vi "RT-Twosetup.vi"() -> ()   [LabVIEW 2015]
uses:
  <vilib>/Platform/TimedLoop/XDataNode/timing_clust.ctl
  <vilib>/Platform/TimedLoop/XDataNode/nitl_modes.ctl
  <vilib>/Platform/TimedLoop/XDataNode/wakeup.ctl
  <vilib>/Analysis/8numeric.llb/1D Numeric Integration.vi
  <vilib>/FPGAPlugInAG/myRIO-1900/niLvFpga_Open_myRIO-1900.vi
  <vilib>/rvi/interface/common/dynamic/niFpgaDynamicAddResources.vi
  <vilib>/Utility/error.llb/Error Cluster From Error Code.vi
  <vilib>/rvi/errors/niLvFpgaAdjustHostInterfaceError.vi
  <vilib>/RVI Host/nirviSupport.llb/nirviErrorClusterFromErrorCode.vi
  <vilib>/Analysis/3filter.llb/Butterworth Filter (DBL).vi
  <vilib>/FPGAPlugInAG/Dynamic/niLvFpga_Close_Dynamic.vi
  <vilib>/rvi/interface/nirviOpenFPGA/nirviOpenFPGA.xnode
  Ruichen Nov 5/FPGA Bitfiles/RuichenNov5_FPGATarget_FPGAWithLasertwo_aS1jXxUkL+g.lvbitx
  Ruichen Nov 5/FPGA_With Laser_twosetup_Jun15.vi
  <vilib>/rvi/interface/nirviReadWriteControl/nirviReadWriteControl.xnode
  <vilib>/Platform/TimedLoop/XDataNode/XDataNode.xnode
  <vilib>/rvi/interface/nirviMethod/nirviMethod.xnode
  <vilib>/rvi/interface/nirviCloseFPGA/nirviCloseFPGA.xnode
  NiFpgaLv.dll
  <vilib>/rvi/interface/Simulation/niFpgaSimulationCallBeginRW.vi
  <vilib>/rvi/interface/nirviMethod/StockFPGA_InlinedMethodWaitForSingleIRQ.vi
  <vilib>/FPGAPlugInAG/Dynamic/niLvFpga_WaitOnIrq_Dynamic.vi
  <vilib>/FPGAPlugInAG/Dynamic/niLvFpga_ReadFifo_Dynamic.vi
  <vilib>/rvi/errors/niLvFpgaMergeErrorWithErrorCode.vi
  <vilib>/FPGAPlugInAG/Dynamic/niLvFpga_AcknowledgeIrq_Dynamic.vi
  <vilib>/Analysis/NI_AALBase.lvlib
  <vilib>/Platform/TimedLoop/XDataNode/XDNodeRunTimeDep.lvlib
  <vilib>/Analysis/NI_AALPro.lvlib
  <vilib>/Analysis/NI_AAL_SigProc.lvlib
panel:
  in  "Gender 2":string="F"
  in  "Date 2":string="2015Aug1"
  in  "Fly # 2":i32=332
  in  "Filename Code 2":string="E1"
  in  "IRQ Bit (0-31) 2":u8
  in  "IRQ Bit (0-31)":u8
  in  "Double number of pixels to take per frame 2":u16=1536
  in  "Half-clocks between frames/Trigger frequency (us) 2":u16=1600
  in  "Half-clock time/FPGA loop timer(us) 2":u32=16
  in  "Gender":string="F"
  out "Raw Data":u16[](graph)=[289, 309, 323, 336, 353, 368, 382, 397, 412, 422, 437, 450, 463, 474, 485, 495, 506, 514, 526, 531, 540, 545, 552, 557, 563, 564, 568, 572, 575, 577, 580, 586, 587, 587, 592, 593, 596, 599, 601, 605, 607, 610, 611, 613, 618, 621, 625, 628, 629, 635, 636, 640, 643, 646, 649, 654, 656, 658, 660, 661, 664, 665, 669, 669, 673, 672, 674, 675, 677, 678, 681, 683, 684, 684, 686, 688, 688, 691, 691, 693, 694, 695, 697, 697, 699, 701, 702, 704, 709, 709, 711, 711, 713, 717, 721, 723, 726, 724, 728, 732, 734, 735, 738, 740, 743, 746, 750, 753, 754, 760, 763, 765, 769, 773, 774, 774, 774, 775, 774, 775, 775, 774, 776, 779, 780, 783, 781, 767, 792, 814, 820, 815, 817, 814, 815, 814, 814, 811, 810, 809, 807, 804, 802, 805, 803, 801, 801, 798, 799, 797, 797, 797, 797, 794, 795, 792, 791, 794, 791, 791, 792, 790, 790, 790, 789, 790, 790, 791, 792, 790, 792, 794, 793, 793, 795, 798, 796, 798, 797, 798, 799, 799, 801, 805, 803, 804, 804, 807, 808, 808, 811, 812, 815, 814, 816, 820, 819, 820, 822, 821, 823, 824, 823, 822, 822, 824, 825, 826, 826, 824, 827, 827, 828, 830, 830, 831, 830, 830, 828, 824, 820, 821, 817, 813, 813, 809, 807, 808, 805, 804, 802, 798, 798, 796, 795, 794, 793, 793, 791, 790, 791, 792, 788, 790, 789, 785, 787, 788, 788, 787, 788, 789, 789, 791, 793, 798, 722, 728, 740, 741, 746, 747, 750, 748, 753, 752, 757, 758, 761, 762, 767, 768, 768, 770, 775, 775, 776, 776, 781, 781, 785, 784, 787, 788, 792, 792, 794, 793, 798, 796, 795, 799, 800, 798, 799, 796, 797, 798, 802, 800, 805, 803, 806, 804, 808, 805, 810, 809, 812, 807, 808, 808, 812, 805, 806, 800, 803, 796, 798, 796, 800, 796, 798, 798, 800, 798, 800, 797, 799, 795, 794, 792, 793, 788, 789, 785, 788, 781, 785, 782, 785, 781, 782, 776, 778, 774, 772, 769, 770, 767, 769, 767, 764, 755, 755, 747, 747, 744, 743, 737, 737, 732, 732, 729, 728, 724, 723, 721, 720, 716, 718, 716, 717, 715, 721, 722, 724, 719, 718, 714, 715, 709, 710, 697, 718, 722, 731, 731, 727, 725, 722, 720, 718, 719, 718, 716, 714, 710, 705, 705, 703, 706, 704, 707, 708, 710, 712, 718, 720, 725, 726, 725, 728, 728, 724, 728, 726, 728, 725, 730, 732, 736, 735, 737, 734, 738, 737, 741, 742, 746, 743, 749, 747, 746, 745, 744, 743, 744, 746, 745, 747, 749, 748, 752, 754, 751, 752, 752, 749, 748, 748, 751, 752, 757, 758, 757, 757, 755, 756, 755, 753, 752, 749, 748, 746, 746, 744, 746, 744, 743, 739, 739, 740, 736, 735, 736, 733, 736, 737, 740, 736, 732, 729, 729, 726, 721, 716, 719, 717, 716, 713, 711, 706, 704, 699, 701, 698, 697, 697, 695, 692, 691, 687, 690, 684, 681, 679, 680, 674, 674, 668, 661, 690, 692, 694, 694, 692, 691, 692, 696, 694, 692, 694, 689, 691, 688, 690, 688, 689, 688, 690, 689, 688, 689, 689, 687, 689, 689, 690, 688, 689, 686, 687, 686, 685, 684, 683, 682, 683, 682, 682, 681, 681, 677, 677, 676, 677, 675, 674, 675, 674, 673, 670, 669, 670, 667, 667, 665, 664, 661, 659, 655, 656, 654, 655, 653, 651, 645, 643, 641, 642, 639, 638, 636, 637, 630, 630, 628, 627, 624, 623, 621, 620, 617, 616, 615, 614, 610, 610, 609, 606, 604, 606, 605, 604, 600, 600, 599, 598, 599, 600, 595, 597, 596, 597, 595, 595, 598, 598, 598, 599, 596, 593, 595, 597, 595, 597, 596, 596, 595, 599, 597, 596, 594, 594, 593, 592, 590, 593, 595, 638, 613, 615, 619, 622, 620, 622, 619, 622, 618, 619, 618, 621, 619, 621, 618, 622, 618, 618, 616, 615, 616, 617, 616, 621, 616, 618, 613, 615, 614, 612, 612, 615, 607, 610, 610, 610, 609, 610, 606, 607, 603, 604, 601, 601, 600, 604, 598, 600, 596, 599, 598, 600, 597, 598, 596, 597, 593, 595, 593, 597, 593, 595, 592, 593, 589, 591, 587, 589, 582, 585, 581, 582, 578, 581, 576, 573, 573, 570, 568, 570, 566, 565, 563, 563, 561, 558, 556, 557, 553, 550, 547, 545, 544, 540, 537, 537, 531, 529, 522, 523, 515, 514, 509, 506, 498, 493, 488, 482, 475, 468, 458, 454, 442, 436, 424, 419, 406, 397, 386, 378, 364, 353, 340, 330, 317, 308, 293]
  in  "FIFO Timeout setting (ms)":i32=5000
  out "Elements going into FIFO":u32=768
  in  "Wait on IRQ Timeout (ms)":i32=100
  in  "Stop LED illumination switch (permanant)":bool
  in  "sampling freq: fs":dbl=1000.0 format="%0.2f"
  in  "high cutoff freq: fh":dbl=400.0 format="%0.2f"
  in  "low cutoff freq: fl":dbl=40.0 format="%0.4f"
  in  "order":i32=3
  out "max index(es) of difference":i32=576
  in  "Threshhold position filter":i32=25
  out "Fly real-time location":dbl(graph)=575.5038458695241
  in  "Fly presence?":bool=TRUE
  in  "threshold 3":dbl=5.0
  out "slope/fly moving speed":dbl(graph)=2.647982912649468
  out "Fly real-time location/center mass":dbl(graph)=575.5038458695241
  in  "peaks/valleys":enum32{"Peaks", "Valleys"}(ring)
  in  "threshold":dbl format="%0.2f"
  out "Laser ON/OFF?":i16(graph)=1
  in  "Laser current control":u16=583
  in  "Laser current control 2":u16=629
  out "peak":i32(graph)=579
  in  "sampling freq: fs 1(2)":dbl=1000.0 format="%0.2f"
  in  "low cutoff freq: fl 1(2)":dbl=40.0 format="%0.4f"
  in  "order 1(2)":i32=3
  in  "Wait on IRQ Timeout (ms) 2":i32=100
  out "Raw Data 2":u16[](graph)=[263, 286, 311, 317, 343, 351, 376, 380, 406, 412, 436, 442, 466, 470, 490, 491, 513, 517, 533, 535, 551, 550, 570, 565, 584, 584, 596, 593, 610, 602, 616, 613, 625, 618, 629, 622, 634, 629, 640, 632, 641, 635, 645, 638, 651, 643, 653, 646, 656, 647, 658, 648, 659, 650, 660, 653, 665, 655, 667, 660, 673, 664, 674, 665, 678, 669, 683, 672, 681, 672, 684, 674, 684, 679, 687, 680, 692, 684, 697, 686, 699, 689, 703, 693, 706, 698, 711, 701, 710, 703, 717, 709, 718, 708, 719, 711, 725, 713, 723, 717, 731, 720, 730, 724, 737, 725, 737, 726, 738, 728, 737, 728, 741, 731, 741, 731, 736, 729, 737, 727, 737, 724, 734, 724, 730, 717, 721, 709, 709, 713, 719, 715, 721, 720, 724, 720, 727, 723, 726, 722, 730, 725, 727, 723, 725, 715, 721, 714, 719, 710, 715, 708, 715, 708, 711, 705, 712, 704, 707, 701, 704, 698, 705, 693, 698, 691, 696, 692, 693, 687, 691, 686, 694, 685, 693, 687, 692, 687, 692, 687, 690, 686, 692, 689, 694, 687, 692, 686, 694, 688, 692, 690, 697, 689, 699, 693, 699, 697, 704, 702, 709, 700, 709, 703, 708, 708, 713, 711, 720, 714, 720, 717, 722, 716, 722, 722, 729, 721, 728, 722, 729, 721, 727, 727, 730, 724, 730, 723, 728, 724, 730, 727, 730, 728, 734, 729, 736, 732, 741, 734, 745, 738, 748, 744, 750, 750, 757, 752, 760, 748, 757, 756, 761, 756, 753, 739, 782, 791, 792, 790, 786, 786, 786, 788, 786, 784, 785, 785, 786, 785, 786, 786, 786, 786, 789, 790, 793, 792, 796, 796, 799, 801, 801, 802, 806, 806, 806, 805, 806, 809, 811, 814, 818, 818, 823, 826, 827, 829, 831, 832, 835, 835, 837, 839, 839, 840, 843, 842, 843, 840, 840, 841, 841, 836, 836, 833, 832, 829, 826, 827, 826, 822, 824, 820, 817, 817, 817, 814, 816, 813, 813, 809, 807, 802, 802, 800, 797, 796, 799, 797, 798, 796, 797, 796, 801, 801, 803, 805, 809, 809, 809, 815, 812, 817, 816, 818, 822, 823, 824, 827, 826, 827, 832, 831, 832, 833, 834, 832, 830, 828, 831, 829, 827, 828, 827, 826, 827, 826, 826, 825, 823, 826, 827, 819, 808, 818, 814, 812, 802, 801, 796, 796, 790, 790, 786, 789, 784, 785, 781, 786, 782, 780, 777, 780, 777, 779, 776, 780, 775, 777, 775, 777, 769, 770, 767, 765, 760, 761, 756, 759, 753, 753, 748, 748, 743, 744, 739, 741, 737, 740, 737, 739, 731, 728, 726, 726, 720, 722, 716, 718, 713, 714, 708, 707, 703, 701, 698, 698, 695, 695, 692, 693, 687, 688, 685, 689, 685, 686, 682, 685, 684, 686, 684, 685, 682, 682, 680, 681, 679, 680, 677, 680, 677, 678, 678, 680, 677, 681, 679, 682, 679, 682, 682, 682, 681, 686, 684, 689, 690, 691, 690, 694, 692, 693, 694, 699, 696, 700, 698, 703, 702, 705, 704, 707, 706, 708, 706, 711, 708, 713, 713, 720, 663, 668, 673, 668, 674, 671, 673, 671, 675, 672, 674, 671, 674, 666, 671, 666, 669, 663, 667, 661, 666, 660, 662, 657, 658, 656, 655, 651, 655, 650, 653, 648, 649, 646, 648, 643, 646, 639, 646, 643, 644, 641, 643, 638, 643, 640, 642, 640, 646, 642, 645, 642, 647, 644, 645, 645, 648, 643, 649, 645, 646, 647, 650, 647, 647, 648, 650, 647, 650, 650, 653, 648, 653, 650, 654, 653, 657, 651, 656, 654, 657, 655, 659, 655, 659, 657, 659, 657, 660, 656, 660, 658, 663, 661, 664, 659, 665, 658, 665, 664, 668, 663, 668, 666, 671, 668, 673, 669, 671, 669, 675, 673, 675, 671, 677, 675, 676, 675, 677, 675, 678, 677, 677, 674, 679, 673, 671, 666, 670, 685, 676, 687, 678, 689, 680, 693, 681, 689, 679, 688, 678, 689, 677, 689, 677, 688, 674, 687, 674, 681, 674, 683, 671, 682, 672, 680, 668, 679, 666, 679, 667, 675, 663, 674, 663, 671, 661, 670, 662, 671, 660, 671, 659, 666, 654, 664, 651, 660, 649, 662, 651, 661, 650, 661, 651, 662, 650, 660, 654, 660, 654, 664, 653, 662, 657, 662, 653, 666, 652, 660, 656, 665, 653, 667, 657, 661, 652, 661, 646, 658, 646, 655, 642, 640, 614, 624, 630, 637, 629, 636, 625, 635, 624, 627, 617, 621, 611, 616, 604, 610, 596, 601, 587, 593, 579, 581, 566, 570, 554, 555, 537, 535, 515, 514, 494, 487, 467, 457, 437, 429, 406, 395, 375, 362, 339, 330]
  in  "FIFO Timeout setting (ms) 2":i32=5000
  in  "IRQ Number(s)":i32
  in  "high cutoff freq: fh 2(2)":dbl=400.0 format="%0.2f"
  in  "high cutoff freq: fh 2":dbl=400.0 format="%0.2f"
  in  "threshold 2":dbl=5.0
  out "Subtraction-10 frames average 2":dbl[](graph)=[-0.00376082484141181, -0.022873117346732395, -0.07050720237291398, -0.1540346374735344, -0.2738381122413475, -0.4232374215403344, -0.5915356082774301, -0.7649563748596452, -0.9279827571524178, -1.0689098028697672, -1.1818944407352858, -1.266468515907346, -1.3239301795845555, -1.3537298053317928, -1.3535024688465405, -1.3236736048293158, -1.2699765892033446, -1.196103151819737, -1.103481168748181, -0.9966608194463829, -0.8808932741469696, -0.7588132471338049, -0.6319358272774014, -0.5061901508981533, -0.389606531794253, -0.28341498123065917, -0.18402265448368677, -0.0895595758834902, -0.0008756313510866129, 0.07639693426695328, 0.133619958700495, 0.16938552040951854, 0.1903441584835061, 0.1997469061336739, 0.19643994001825865, 0.1826729540490901, 0.1615768169464919, 0.13332481872660476, 0.10013796877874595, 0.06705342198095826, 0.03830291760632126, 0.01812410505187573, 0.011040299585847513, 0.015678182445511897, 0.02081490655012259, 0.014702139724543097, -0.007694751105500634, -0.0446452896519642, -0.08670643610239012, -0.1277979715847761, -0.17541766675378068, -0.23978598654637842, -0.32345963765313057, -0.4259229913641579, -0.5469672931754658, -0.6838484323216937, -0.8312503325824077, -0.9825087887632742, -1.12867925796915, -1.2633122581370897, -1.388947954682801, -1.5076359517362217, -1.6119373954936247, -1.6958213101732502, -1.7616620044088953, -1.812529334752833, -1.8486816415803766, -1.8719732738452068, -1.8847414740848745, -1.8859257219554215, -1.8743803959335448, -1.849487948127098, -1.808197256512122, -1.7466329724933511, -1.6611929495136815, -1.5482907626170368, -1.4067508767371109, -1.238889497628028, -1.0483066610520457, -0.8410518480858593, -0.6285318110483396, -0.42486535833667716, -0.24156551097017567, -0.08552176857086577, 0.03983825028626295, 0.13356818406741786, 0.19717522191258308, 0.23278936634599218, 0.24150276211340116, 0.22730699422553458, 0.19899536076779312, 0.16605439722890952, 0.13693874170986747, 0.11613849442096771, 0.10209305304397168, 0.0912139405376808, 0.07866812938458467, 0.057773934292369024, 0.024749420335167242, -0.017230893747750352, -0.061913083640327604, -0.10784179345245254, -0.15830391148879083, -0.2143877330715396, -0.276778621610512, -0.3528272911072182, -0.44913895643011553, -0.5595612194406266, -0.6704730509504452, -0.7745604578629908, -0.8731593145809257, -0.9701116617591585, -1.069496797609171, -1.1730905057698047, -1.2777684274273855, -1.379916659751327, -1.4814777777037755, -1.588047949586358, -1.6986990178288548, -1.802015100812946, -1.8826514219000368, -1.9293015986204978, -1.9402172728964677, -1.9208181943344855, -1.8769697908343117, -1.8134710392918705, -1.733963461335194, -1.638587583967085, -1.523674399142967, -1.386346749941397, -1.2291419386239086, -1.0583515986225247, -0.8836878074942338, -0.7187385558367253, -0.5738173894502159, -0.45542305080593687, -0.3701037445479088, -0.317616230630637, -0.28930799633113535, -0.27602190239510177, -0.27115275142298206, -0.2717125476718229, -0.2774216061797233, -0.2867771895763348, -0.2981017950239787, -0.31178072131091655, -0.32608937059191756, -0.3353603508176363, -0.3357385368030959, -0.32681389734130667, -0.31103915970614604, -0.2946481407676892, -0.2807293154814101, -0.26451167744311843, -0.2407094121827115, -0.211050327886528, -0.1837625411526074, -0.16707239135883667, -0.16611371302420752, -0.18394775224048487, -0.21857278595226554, -0.2612999759586515, -0.30543475903423317, -0.35471060592599035, -0.41718212157458284, -0.49648878909719873, -0.5921132750867147, -0.7022809147875497, -0.825066949533824, -0.9576931927650932, -1.0951203986321776, -1.2307248788941316, -1.3591314014615774, -1.47693568696294, -1.5800230024344128, -1.6623793299744725, -1.719229265770608, -1.748876372099362, -1.7497891567424408, -1.7174342402814031, -1.6478702779804903, -1.5444577832306738, -1.4177442273018168, -1.280676739644643, -1.1434442501256068, -1.0128407801542985, -0.8932081460963361, -0.7801274495106644, -0.6621789141760148, -0.5372155137010306, -0.416657868348343, -0.31038743641522437, -0.21810966155455125, -0.13683865247976046, -0.06492287746215691, 0.0011107561638208675, 0.061355697754530085, 0.11016677649880281, 0.14364453618861886, 0.15949885750470377, 0.15778587381061385, 0.14364154198124413, 0.1227551498373353, 0.10305638615350414, 0.09370311790900986, 0.09640586325429953, 0.1068123624264574, 0.12066322960728416, 0.13426468214309775, 0.1405369170182361, 0.13235826724673255, 0.11110335132503889, 0.08002488785588409, 0.03737629353642087, -0.018637808401881423, -0.08700059597261785, -0.16054846664987324, -0.23088586621000848, -0.3000360164872003, -0.3758296150061959, -0.46236970350596185, -0.5587974369384311, -0.660898934677404, -0.7660448460774516, -0.8729260247349662, -0.9767431951499936, -1.0748340624377097, -1.1705342177905071, -1.2675451899107062, -1.3683321205241692, -1.4704192038160353, -1.5635451916548424, -1.6386695835358795, -1.693256497574253, -1.7277824542414204, -1.7420870638626291, -1.7322894565104652, -1.6933942206714316, -1.624322634361078, -1.528407672990961, -1.4124576261429136, -1.2832747700098635, -1.1468778581044203, -1.01116382986234, -0.8850483573844115, -0.7788370742693432, -0.7004306032861471, -0.6487688874247476, -0.6180821163401873, -0.6030060400253653, -0.5959037847747308, -0.5875920612480976, -0.5741500995988539, -0.5582423972416175, -0.5439443648942461, -0.5328073893976564, -0.5232639086012941, -0.5146518432728002, -0.5090998137587567, -0.5065819566515576, -0.5038548193517427, -0.5005796544437178, -0.5002479504085452, -0.5014087461956691, -0.495040446888778, -0.4727119725533419, -0.43125038067469823, -0.3715074504347726, -0.3008338507948245, -0.23340738667639166, -0.17755289527540508, -0.13118575191904772, -0.09305928514965348, -0.06698996053837801, -0.058563480577701686, -0.07181350001125919, -0.10793573000127399, -0.1689908845929966, -0.25596119116887905, -0.3615529177179252, -0.4739173690044841, -0.5852687043626082, -0.6925790166307004, -0.7935196446787861, -0.8831899624548932, -0.9549489633523359, -1.0053936034989386, -1.034287291347867, -1.0417180668143775, -1.0307381755818692, -1.0022200877051664, -0.9517839735970008, -0.8847816574868836, -0.8203025453751498, -0.7740566015333439, -0.7450169971868286, -0.7211422986874927, -0.695447400598044, -0.6662409751476156, -0.6267691166515336, -0.5709534536668012, -0.5062730580488137, -0.4485965248982422, -0.4042914265127707, -0.36774155042836065, -0.3351346131083027, -0.31079122745476945, -0.29983578466573796, -0.29704845614316383, -0.28648550431823483, -0.2560797219170984, -0.207191797964983, -0.15002634485714278, -0.0941146339452417, -0.04141132907327572, 0.00732382089288372, 0.04527845665160592, 0.06729656650068232, 0.07648330949975393, 0.08064998018063296, 0.08649692634618564, 0.09611867663977593, 0.10592138239814952, 0.11046023397899403, 0.10860213666725135, 0.10263107983657813, 0.0951675648597761, 0.08755686894783427, 0.07727335537096702, 0.06050473908625864, 0.03858170245257776, 0.019016774014489195, 0.006217689491663469, -0.004829580964054308, -0.02187946084338151, -0.05041171001791412, -0.09262496242405108, -0.14569587160812036, -0.20561733612433442, -0.27547542848413525, -0.364110224847606, -0.4722816750400199, -0.5869343272139628, -0.6915599909578858, -0.7801941030271669, -0.856503792838089, -0.9183491975010316, -0.9560750231796934, -0.9649909582222269, -0.9473373048466116, -0.9066887049224265, -0.846911733740316, -0.7719296640245625, -0.6853692031922703, -0.5898590863699504, -0.4838455537247155, -0.3599201532402052, -0.20883433515499233, -0.028636455612853818, 0.16983555954076301, 0.36973615220851197, 0.5591901850809423, 0.733067351126909, 0.8883202563929481, 1.0221095816515888, 1.1375825701281228, 1.2453575621607862, 1.3512137702495255, 1.452792799750593, 1.5477941475302321, 1.6378527323460585, 1.729241387236583, 1.824010182307176, 1.9170375875927546, 2.0097098629114285, 2.108943976314938, 2.215027391713627, 2.3230331304401033, 2.429548985942421, 2.5355477549070238, 2.6464477153608295, 2.7702576533997356, 2.9131377100839217, 3.073678261038705, 3.244552757581614, 3.4204261801800553, 3.602300947020557, 3.794056055282762, 3.996592870664724, 4.2075413784439135, 4.424550583066579, 4.648714283923216, 4.880038620061748, 5.110417378684536, 5.330743067375148, 5.538073955911634, 5.732219184144099, 5.918123480846642, 6.110372500362169, 6.327000370177558, 6.583321692370052, 6.8906167476800295, 7.255257453715437, 7.68027948763792, 8.166604119726658, 8.712237640790278, 9.313494022979661, 9.964056663838145, 10.654892015352061, 11.378324058152502, 12.127175033359443, 12.895230216622453, 13.678603979404247, 14.474046709861591, 15.279470627616204, 16.090738173396232, 16.902158085596497, 17.714679222144923, 18.53315978571027, 19.358338660702593, 20.187216642994212, 21.01194814379528, 21.82222777219512, 22.61602191722952, 23.400763975924672, 24.184327855534672, 24.971785834110076, 25.768504552430322, 26.57753306161372, 27.396165036084163, 28.221325795503553, 29.049922125954453, 29.873139470742423, 30.679593833577684, 31.4609081749663, 32.212712825571906, 32.933051665490176, 33.619965819210464, 34.271625765457, 34.8890859732, 35.478764581385875, 36.04756436585725, 36.596346257203344, 37.12343236422261, 37.626822539780484, 38.105588462364175, 38.56611234545378, 39.01491060125615, 39.44715283367774, 39.853534247824754, 40.2310712889892, 40.57888757186952, 40.892349191698884, 41.16933128074967, 41.414110482177485, 41.63342646341003, 41.83363247239842, 42.018303435619615, 42.18872817010225, 42.34408970348531, 42.47754928608451, 42.58236130365064, 42.65971748760769, 42.713644181365986, 42.74525521883325, 42.748753326527726, 42.713333823695294, 42.63449439250565, 42.51642043459606, 42.364574210563276, 42.17993378111193, 41.9556039072654, 41.68122828230601, 41.35096432259596, 40.962156501385, 40.512861591872834, 40.00642312420001, 39.451821047297614, 38.85541134665982, 38.2173537339134, 37.53692246110689, 36.813455534636056, 36.044893402993836, 35.2315962369416, 34.377010210901396, 33.484762597643936, 32.557001280199344, 31.593345539691676, 30.589708555804926, 29.540802457970848, 28.44559042107734, 27.307847611971, 26.133341471138614, 24.926617171868227, 23.690992747103518, 22.429412137004675, 21.141197570572455, 19.823253456474465, 18.472937657505387, 17.085399392921254, 15.65521449602104, 14.180158509493307, 12.661336060618844, 11.104659392517387, 9.520123594285872, 7.917416475572328, 6.3027034652523515, 4.682263341486394, 3.0660056719976527, 1.4612989176075901, -0.13139771239858228, -1.7123880812285628, -3.2751905848703613, -4.808174608992262, -6.297740620268804, -7.7271473935905215, -9.081790002488592, -10.356133616169028, -11.554151135074896, -12.685676557678587, -13.758362721441806, -14.77575035037717, -15.74255078525408, -16.666415835412305, -17.556443863742437, -18.41732773000568, -19.24820734880522, -20.050495274673978, -20.828771105634228, -21.584545223346325, -22.314638216729037, -23.014595247144705, -23.680923116221063, -24.31176928795577, -24.907986296652496, -25.472415693796478, -26.006884426442767, -26.509208132203728, -26.97444501410167, -27.398008728417842, -27.77647645316585, -28.110048905215564, -28.40385378205497, -28.668367565302646, -28.917474740737617, -29.15755911012913, -29.384038238726703, -29.589748868420692, -29.76924544606401, -29.918328165454806, -30.036045206361063, -30.12937311357554, -30.208794995708473, -30.277806917764497, -30.332825573826625, -30.37151391821005, -30.39725409536827, -30.412656938396555, -30.413956258287868, -30.39735109458483, -30.36367151738291, -30.31652542478745, -30.261502338976612, -30.204184510465918, -30.14871940232551, -30.097352108584346, -30.047784376662662, -29.993910764165935, -29.92747733828788, -29.837193104698244, -29.711437717836816, -29.54242404233223, -29.327043752160268, -29.067452267851255, -28.771375859675317, -28.448234996158785, -28.103706205315063, -27.739064252815734, -27.354938800750066, -26.95410602345842, -26.539649974551562, -26.111747453405904, -25.670224697083718, -25.216450073218372, -24.750712831780145, -24.272616690419394, -23.78091619861165, -23.2753928522925, -22.761343164505224, -22.244816004276867, -21.72786594335049, -21.21417978538097, -20.71071063748661, -20.222789714979534, -19.753607797772467, -19.301867144951565, -18.86158004391697, -18.43123343688248, -18.0143840109354, -17.61041314054533, -17.212941896681723, -16.81748076620043, -16.426715057545632, -16.04531884239273, -15.675168217712752, -15.31754391861577, -14.974344529674788, -14.649051560367349, -14.343674232203869, -14.054821664391083, -13.777985913802734, -13.508879451605642, -13.242082589313352, -12.97275008446546, -12.696082444150797, -12.409256262549752, -12.112442043542092, -11.807571599785787, -11.503046705893926, -11.21227271056884, -10.942267303072779, -10.691045639568582, -10.457244745998056, -10.244016574854548, -10.051518531924048, -9.87061623279275, -9.685855538473072, -9.483993882353875, -9.258017630799372, -9.007354147311343, -8.735371178658298, -8.443853548820478, -8.134648990461866, -7.813610715699731, -7.487832383457061, -7.162206460899759, -6.839682212706416, -6.5231322433607275, -6.217234714158364, -5.9289138057546955, -5.6619823667673765, -5.412579923126114, -5.173133122357569, -4.938792509122974, -4.710971908054537, -4.495125783066928, -4.29488827490601, -4.109283009973048, -3.9339855929532987, -3.764175462971437, -3.5958951815680615, -3.4233935393454833, -3.2394830683479725, -3.044598200547575, -2.8492028556439815, -2.6649359565198165, -2.498850507216461, -2.351994989596593, -2.2200416457008263, -2.097354106644154, -1.9816741134997693, -1.8733763519173783, -1.7695976868323733, -1.6661986077487314, -1.5661702552726366, -1.4769612407021504, -1.4022436450621427, -1.3413180588193816, -1.2916765418291913, -1.2507505025842343, -1.217944653778875, -1.1955330573680045, -1.1903154857303306, -1.2136419659976456, -1.2738107603937543, -1.3724390980490855, -1.507885962350215, -1.6763896973186003, -1.8711191364837378, -2.080717766297735, -2.2916512250453622, -2.4928182004627035, -2.6755849779817424, -2.831334628203854, -2.949936208348438, -3.018931043968457, -3.0298384774615834, -2.986716161838226, -2.9013396647233263, -2.783940766628996, -2.6407616499493893, -2.4767875282446816, -2.3001157310922586, -2.119033148960194, -1.9363683567416965, -1.753289795851237, -1.5770678151434212, -1.4153899237661798, -1.26683678826652, -1.1294693920602856, -1.0081263553709296, -0.9063889971623248, -0.8232096500754797, -0.7569594986576507, -0.7051277446235275, -0.6609626172844825, -0.616778811364658, -0.5706830022030382, -0.5238540351402355, -0.47530875658731897, -0.42318424546559685, -0.3665577694236487, -0.30756730783451597, -0.252067836451747, -0.20443771113836468, -0.16562044808556212, -0.13522655672247405, -0.11042486682504797, -0.08882597340265397, -0.07538417283274809, -0.07845722411255573, -0.09901308223776047, -0.13026897814939803, -0.167681023057152, -0.216864963214016, -0.2876508278340629, -0.3808876121771616, -0.48834768637964654, -0.6016077538625505, -0.7144036890985765, -0.8233041134798268, -0.9286804831666096, -1.0311741155510397, -1.1278050469591983, -1.21391289217402, -1.2898718155112867, -1.3623238656310392, -1.4395570531631365, -1.525478966414576, -1.6149241061519883, -1.6997189909924915, -1.778996289119347, -1.856765587267083, -1.9288164466428759, -1.9803244023449569, -1.9995236930547802, -1.9845766247298668, -1.9402420483774412, -1.8734661368225516, -1.7868241836145662, -1.678066806724053, -1.5470606760189267, -1.3999431271868326, -1.2465844830197161, -1.0965471302864371, -0.9576500186057677, -0.8342253141905895, -0.7249247595230404, -0.6233497672777235, -0.5244663209042256, -0.43092374400637523, -0.34844608354784923, -0.27579555458255645, -0.205640126840743, -0.13310105896139204, -0.05745891472761272, 0.020014086631217332, 0.09599766173239417]
  out "Integral of fly movement 2":dbl(graph)=79328.12499999988
  out "Fly real-time location/center mass 2":dbl(graph)=449.3915049700411
  in  "Fly presence? 2":bool=TRUE
  in  "Threshhold position filter 2":i32=25
  out "Subtraction-10 frames average":dbl[](graph)=[-0.00017411226117643476, -0.0013055996545707524, -0.0035903395574269233, -0.006140247965520452, -0.00923276869863789, -0.014513306411590609, -0.024099157253657542, -0.039967772567530944, -0.06357541427301813, -0.09583108984311303, -0.13590150060754386, -0.18222853004778936, -0.23497195652311498, -0.29627873859507925, -0.36762235578800867, -0.4458020453794083, -0.5236122536857144, -0.5933213778936878, -0.6504861464069396, -0.6979211584984373, -0.7411188663256683, -0.7815085830005122, -0.8183155891766691, -0.8521623071897098, -0.8841462084502619, -0.9134837246856654, -0.9369680551554314, -0.9497776612221199, -0.9486128151755009, -0.9320974118038038, -0.8980743313625289, -0.8467722222222394, -0.7831903740903514, -0.7091535422572258, -0.6191326605534678, -0.5096162410693632, -0.38445407095366013, -0.25038829684524394, -0.11278151470849465, 0.027599357220651342, 0.17105909212912457, 0.31047378816969246, 0.43477068100652727, 0.5404159738124296, 0.6300372451091932, 0.7028022222295014, 0.755728962675972, 0.7909826153091774, 0.8173402496662823, 0.8426901249940745, 0.8646090232247912, 0.8743645244461501, 0.8649039706505928, 0.8319565719228973, 0.7750164581136465, 0.6955035375961216, 0.595281511328262, 0.47813554162155286, 0.34852361101846857, 0.21192255735328513, 0.07591841420380419, -0.05221188114593133, -0.1699837988889325, -0.28130279822899423, -0.39034428199093896, -0.4976048670003517, -0.600986712631866, -0.6958495060431942, -0.776729298015907, -0.8400889448088852, -0.886367229474972, -0.9177076114860692, -0.9344855611862907, -0.9368525887383509, -0.9256879281616348, -0.9041394572607666, -0.8777818783736817, -0.8490193014663585, -0.8164059788053225, -0.7777460019674792, -0.7306702277622628, -0.6758164055484195, -0.6196815773574544, -0.5696251531398948, -0.5294590057849148, -0.5036816824661907, -0.4967820810630079, -0.5075400503507222, -0.5296116117376369, -0.5541794866502316, -0.572591220019981, -0.5770013677344076, -0.5579969792703307, -0.5077796604374197, -0.42865181791737544, -0.33090735363867285, -0.22215393525511828, -0.10432496528395577, 0.023095326221807485, 0.15705894844325297, 0.2880394188853618, 0.40439012577347405, 0.4963650319027993, 0.5611047944479498, 0.6048704375837946, 0.6333678585164843, 0.6444899475696537, 0.6328680620173739, 0.5949073615035211, 0.5317088662054599, 0.4484691112083726, 0.35262691347111735, 0.25592435302870753, 0.1677918630477906, 0.08552896387664585, 0.001721814571532223, -0.08465072369990116, -0.16887968342886978, -0.2446520248995666, -0.3085125998395212, -0.36285963309259667, -0.412304954070232, -0.45947045202927694, -0.5043419236517144, -0.5430792956503917, -0.5701392528804239, -0.5823970562876603, -0.5798838911637391, -0.5657644118110517, -0.5445993018003239, -0.5216310512058843, -0.5004822604773764, -0.48152211922137, -0.46657488631796473, -0.45829805549562763, -0.45812891230711617, -0.46688057094727364, -0.4832346439961762, -0.5040900061989401, -0.5246298701963221, -0.5396268618306358, -0.5486879364347477, -0.5553220286350682, -0.5602243690739389, -0.5619992550807327, -0.5616390340191147, -0.5618614340001415, -0.5619878499927449, -0.556044076174116, -0.5375776201240388, -0.5018226807722814, -0.4441251771537087, -0.3609544857301398, -0.2542849281294559, -0.1337061514028871, -0.01077592265797097, 0.10802739138302234, 0.2204702742907546, 0.32334046947867695, 0.41151196363946524, 0.4802339911288074, 0.5261902901839506, 0.5468284379398634, 0.5388710085338079, 0.5013551052040558, 0.4402253796787686, 0.3649945548717722, 0.28453393264954674, 0.20500115403415162, 0.12737052447350872, 0.0491965117891805, -0.033624099556903625, -0.12401511839311359, -0.21772721743544826, -0.30600877804536525, -0.3845380193961243, -0.45271563684577065, -0.5083720110481487, -0.5483993223855057, -0.5692595973559456, -0.5689429763761056, -0.5496008669456361, -0.515240588241775, -0.47411449414621015, -0.43757582550721474, -0.4100771941058324, -0.3912010975889608, -0.3827420386611698, -0.3870110616763467, -0.4048639535633476, -0.43620163141685364, -0.4793177697728358, -0.5289343816851729, -0.5783732084027549, -0.6226483831393546, -0.659195235246784, -0.6900328665239266, -0.717743997948285, -0.7393052243940111, -0.7488387052387162, -0.7410064339076299, -0.7151668280354428, -0.6795465516096135, -0.6411676626175322, -0.5963042174390132, -0.5382989954290448, -0.4642086308424046, -0.3750273950060304, -0.27666264335898244, -0.1726805762033885, -0.061141495920442324, 0.055284462096357824, 0.16923993804278972, 0.2757778422982206, 0.3702189250517674, 0.44567248716703034, 0.4961833944600499, 0.519491459859946, 0.5161197856703529, 0.48925516442404415, 0.4457811453867938, 0.3931640243514122, 0.335508631703314, 0.27666000462165524, 0.22536122034470552, 0.18892461638725597, 0.16561938458101683, 0.14877029060355898, 0.1316923262868149, 0.10936359529509165, 0.07708080345845039, 0.03176571652430371, -0.02126415203944002, -0.07462865099459134, -0.12787029966300012, -0.18232016801891016, -0.23903213138123067, -0.3005074000846957, -0.36721761077858145, -0.4351648227660777, -0.49748480603309386, -0.5504691500712211, -0.5969563855516151, -0.6388566462772594, -0.6732204448166237, -0.6957500128580998, -0.704492654543993, -0.7053606511252234, -0.7068255505670542, -0.7111454456488149, -0.7171014427168811, -0.7204222977914532, -0.7121147912086817, -0.682707841299486, -0.6275912533817392, -0.5508914834780626, -0.4629445080600611, -0.374231847988499, -0.29348756884376326, -0.22608532636693335, -0.1717419914367267, -0.12418215830144208, -0.0759240199102344, -0.023465854733136317, 0.03495613368073635, 0.10364757933210111, 0.186875978170696, 0.28047176945614266, 0.37246623408448487, 0.4537540089905635, 0.5221189090366725, 0.5772629148585383, 0.6195437842721869, 0.6505398797841452, 0.6673383091587535, 0.6621500666273517, 0.6294188669879256, 0.5678884026793507, 0.4776367246700199, 0.3619901254764424, 0.22990267247159088, 0.09066434134522192, -0.04648363107378383, -0.16799140274521498, -0.2619477892108051, -0.3288086467882362, -0.3780169598975864, -0.4147345107790823, -0.4399946988218713, -0.45778196758191586, -0.4728903322312472, -0.48932022274099063, -0.5119453113587404, -0.5438949360668957, -0.5850957300740083, -0.6332562764482668, -0.6817369661192783, -0.7196211852955186, -0.7411725102754282, -0.7520087863705485, -0.7603886734107392, -0.7693352686888594, -0.7780724435008916, -0.7860412698523446, -0.7953131974335302, -0.8093398039386801, -0.8283695763831367, -0.8473220299068974, -0.8630717050367799, -0.8783577081132093, -0.892945116030908, -0.8982166970622634, -0.8843691812454313, -0.8489983341041851, -0.7981453240654648, -0.7378847051244974, -0.6655070232853431, -0.5735742180168014, -0.45708106421106715, -0.31639925961468957, -0.1590737866558735, 0.0033355840614780405, 0.16185921651742433, 0.31258646062391215, 0.452338343404292, 0.5749805575018252, 0.6712888680367465, 0.7315341547033588, 0.7517398814338361, 0.7348880070093617, 0.6857398390731334, 0.6111385134913258, 0.5228723096640573, 0.4318324111699806, 0.34025172401448045, 0.24736937305364776, 0.15784156635128652, 0.07651042206858172, 0.003772883581942832, -0.0629782232996971, -0.1286940081175351, -0.19772726178007713, -0.2713596192561732, -0.34779592456603625, -0.42333992685501454, -0.49628751054437203, -0.5666772253075136, -0.6286643732283865, -0.6728023696181352, -0.6962315973004579, -0.703034713648139, -0.7020136014256354, -0.703404439937798, -0.710015320364523, -0.7156617656943353, -0.7127960782972558, -0.6987305516219793, -0.6767153962682136, -0.6525149153664662, -0.6316849293158644, -0.6187483363957781, -0.6144729279978336, -0.6180486050640402, -0.6330864189293007, -0.6627772041805703, -0.7019166712317585, -0.7393755374665935, -0.765505461453525, -0.7764222036847284, -0.7696638037044172, -0.74111805905735, -0.6910322911182983, -0.623579160676762, -0.5383420920997759, -0.43065265289455934, -0.3002573308746692, -0.15092259425682136, 0.015622110790919387, 0.1946442614540931, 0.3730903109812267, 0.5367123338443216, 0.6790157566567216, 0.7995832395645845, 0.8951896619070442, 0.9608299845005637, 0.9968364468122866, 1.0067579713827326, 0.9912086432745015, 0.9482471263296486, 0.8811804893600276, 0.7989187264121542, 0.7078954125144599, 0.6120374936386584, 0.5141496232828386, 0.4142079445676434, 0.31468652890071547, 0.22211899540161129, 0.1399216579039876, 0.07005059700724892, 0.017247963468361452, -0.015501622682586178, -0.03254984006910774, -0.04612893264658296, -0.06952650175657003, -0.11252353348731638, -0.18040885529329365, -0.2721680628995837, -0.3822515911818568, -0.5017857806819399, -0.6198988731614818, -0.7262369995249518, -0.8111728656936505, -0.8684225357345006, -0.8990058995890593, -0.9075499623628133, -0.8977470496940952, -0.8745268143081815, -0.8441468656929902, -0.8112598244140514, -0.778277057340187, -0.7477741175043585, -0.7252892407870994, -0.7168386207607349, -0.7232909271474866, -0.7365659877890743, -0.7414056214816782, -0.7280969588471254, -0.7004614128383602, -0.6670127989797451, -0.6331576747915737, -0.5977492527834072, -0.5524997568983321, -0.4900541210242786, -0.40608708648086494, -0.29564160282918805, -0.15660928933041263, 0.007186595218111103, 0.18629507602397022, 0.36646272580965705, 0.5332396031733194, 0.6768763941517248, 0.7907893517687489, 0.8712917590344003, 0.922780189304281, 0.9537929539711842, 0.9687394176061441, 0.9693260986597775, 0.9552998439742726, 0.9240374691005266, 0.8771673370192855, 0.8211939500761857, 0.7591571431502234, 0.6926676856627026, 0.6284730370506213, 0.5707184781226731, 0.5152431462804957, 0.45636062097298347, 0.3918646995312176, 0.32210119515646674, 0.24777271899974834, 0.16944111121942207, 0.08427298985578352, -0.013485790267639703, -0.12456713336305435, -0.24399633307965893, -0.3642314265649915, -0.4747812371557585, -0.5646437823813745, -0.6265764327719912, -0.6573275140072035, -0.6558789526974032, -0.6221897569890409, -0.5600029777218457, -0.4804061725317835, -0.3934102515117905, -0.30283676942819754, -0.21228827793009214, -0.12333279093058303, -0.035098823919149306, 0.04911526715647138, 0.12628668299424806, 0.20141522088447067, 0.280948100266101, 0.3626726363188982, 0.4384522788136301, 0.5061083683109453, 0.575375006200826, 0.6582532028795898, 0.7558580451840798, 0.8603507020065457, 0.9653936278157114, 1.0692725123865725, 1.1718470525300688, 1.272738426840291, 1.3709577035007996, 1.4661433723369786, 1.559081041169027, 1.6489409903984935, 1.731769923726097, 1.801486773489075, 1.8537182263756429, 1.8902753234771437, 1.9186485003323326, 1.9460313929763289, 1.97442918741, 2.0056475617894116, 2.0446506904852857, 2.092528372086769, 2.1483396284249947, 2.215650396354458, 2.294876136594476, 2.381207065473582, 2.4748699018686904, 2.579717423360695, 2.698160537409042, 2.8323892111726123, 2.9816208879989032, 3.1442066260393498, 3.324402132118785, 3.5261056451825965, 3.746273498221313, 3.9836396532216556, 4.242440972110447, 4.5259197205480985, 4.834539532183516, 5.168294180188352, 5.52727552599602, 5.907827657991055, 6.304448282685934, 6.717446041575664, 7.150231908029313, 7.603695367024238, 8.077557189762695, 8.569383573295394, 9.073002597804843, 9.586155756115309, 10.116177716337475, 10.674086352879788, 11.269313159769121, 11.907593760086048, 12.58596064564858, 13.293872665342972, 14.021698080945395, 14.760652096041209, 15.498437700869376, 16.22492798636594, 16.939702787230615, 17.653266946601153, 18.381937914543425, 19.134436194857358, 19.902814424794155, 20.67064045169619, 21.424507186952862, 22.15791275844625, 22.872347661912087, 23.573707576768765, 24.264767732228037, 24.940021340560794, 25.588797898169314, 26.202635937391022, 26.776155442184255, 27.306843522461016, 27.79660513139952, 28.250350047289217, 28.672709014652686, 29.064973148731724, 29.42510629441868, 29.751221359110012, 30.04682421891593, 30.319605834762413, 30.57308847323303, 30.80819053733222, 31.03032226851724, 31.244481307843223, 31.44860922606201, 31.633219821591105, 31.785118037096588, 31.894683720978225, 31.95779661586935, 31.971838584533376, 31.93230113062428, 31.83445047092844, 31.679985300967314, 31.47904662556253, 31.240073211247434, 30.9618103917683, 30.641239024952768, 30.281875468623436, 29.889428407606488, 29.465243368494367, 29.010043956957578, 28.52972296658352, 28.029754915590125, 27.509353290472298, 26.96514906445715, 26.39317290784618, 25.788417105068145, 25.149083022013173, 24.476259573025132, 23.768571743932227, 23.025287939120506, 22.251106424242593, 21.450648124554377, 20.622293136463593, 19.761151721111734, 18.865577196239634, 17.940123139596853, 16.990428329916373, 16.018388105591544, 15.026700188156017, 14.01436384300455, 12.97083500677785, 11.889881275078858, 10.77466922188803, 9.628258702052682, 8.454448195724423, 7.265133695016243, 6.076365535034785, 4.893365123282578, 3.7095532614713296, 2.517763517138069, 1.3140267408770159, 0.10309209642734382, -1.097192432889481, -2.267385411930342, -3.3944907621586125, -4.469239206666381, -5.489787294397093, -6.459802537068538, -7.38100261281204, -8.257687685899288, -9.100751446659293, -9.922390196002823, -10.73071732580621, -11.5262653960874, -12.302138094129747, -13.051669492570305, -13.771894442454053, -14.458721932895862, -15.108005691893894, -15.72129731761331, -16.307379747694846, -16.877187908027814, -17.43744317765741, -17.991119943063904, -18.54065018507351, -19.08674531756916, -19.62278622788451, -20.13463627958771, -20.60680191243237, -21.02438534875431, -21.376310849903668, -21.658624268879443, -21.86977992174831, -22.011941620880712, -22.09505301916887, -22.129394797421718, -22.123365749377168, -22.08586833329003, -22.020104554291713, -21.9238000455441, -21.79858267495767, -21.653175725941942, -21.498289904431616, -21.343914968258687, -21.197799477152486, -21.062728377100974, -20.938961251530145, -20.824718023521243, -20.717206642785232, -20.615462348219484, -20.515811184705363, -20.412387296008212, -20.30451311016455, -20.194590015757164, -20.082154952053266, -19.965437180049225, -19.84418363236728, -19.71966080590015, -19.59101651633682, -19.451896747520415, -19.29630570606669, -19.124625370339928, -18.940908553959353, -18.74841398094579, -18.548334850520973, -18.34390884585281, -18.142670376332994, -17.946870545009805, -17.74763036520624, -17.535438988826193, -17.309111329506337, -17.073475808836182, -16.838228485832403, -16.616666753603663, -16.416761917507017, -16.237902387884915, -16.077044504285908, -15.927991530686892, -15.778194878136429, -15.618016239883016, -15.44547675943471, -15.259036731177005, -15.057565030108478, -14.841515625944622, -14.608958358145568, -14.358650294416119, -14.09462865748661, -13.822698270104837, -13.54650548098001, -13.265495449822433, -12.973379194579834, -12.6637392519324, -12.336642526018718, -11.99750459600148, -11.654793828507898, -11.314946313361293, -10.97644226630489, -10.635343587106952, -10.290828574749673, -9.944251504563086, -9.601837487332826, -9.273690255644487, -8.967830376318314, -8.689646700736837, -8.443309094072085, -8.230419468928783, -8.049589622644953, -7.899441492653072, -7.778172513279259, -7.678654073677392, -7.588666634736229, -7.496717485742737, -7.397547046258119, -7.289718378538725, -7.168077924542731, -7.028490811396077, -6.877623118566651, -6.7283616982472125, -6.588994662979143, -6.45961051981716, -6.335907389209561, -6.213871508147667, -6.092452979069016, -5.972482269112145, -5.853392865729774, -5.732945383951386, -5.606896264537465, -5.469907708842971, -5.322011725262907, -5.170622617466721, -5.019133870887847, -4.861231237999979, -4.6918455000478305, -4.51214993000221, -4.324497437985056, -4.131660461805229, -3.9392579288830207, -3.754622884073377, -3.5851706825546588, -3.4381831491227537, -3.3172911818944666, -3.219947302195386, -3.138072117665304, -3.059582753466284, -2.9724515330751533, -2.869044637751715, -2.7454704463662214]
  out "Elements going into FIFO 2":u32=768
  out "peak 2":i32(graph)=455
  out "Locations":dbl[](array[numeric])=[578.761004094259, 639.2528301043833, 668.0679203678199, 696.7815537364846, 725.476037300267, 754.2154459301402]
  out "size(s) 2":i32=7
  out "Peak":dbl=579.0
  out "Locations 2":dbl[](array[numeric])=[464.590182599329, 527.8415122083895, 556.6315016603198, 585.3519264680052, 614.0835380602954, 642.7960329445821, 671.488231054549]
  out "y":dbl
  out "size(s)":i32=6
  out "Peak 2":dbl=455.0
  out "Wait on IRQ Timed Out?":bool
  out "Frame Count":i16=10040
  out "Wait on IRQ Timed Out? 2":bool
  in  "Stop FPGA data acquisition":bool
  in  "high cutoff freq: fh 1(2)":dbl=400.0 format="%0.2f"
  in  "Manual control for laser":bool
  in  "sampling freq: fs 2(2)":dbl=1000.0 format="%0.2f"
  in  "low cutoff freq: fl 2(2)":dbl=40.0 format="%0.4f"
  in  "order 2(2)":i32=3
  in  "sampling freq: fs 2":dbl=1000.0 format="%0.2f"
  in  "low cutoff freq: fl 2":dbl=40.0 format="%0.4f"
  in  "order 2":i32=3
  in  "threshold 4":dbl format="%0.2f"
  in  "peaks/valleys 2":enum32{"Peaks", "Valleys"}(ring)
  out "x/y 2":dbl=449.3915049700411
  out "x/y":dbl=575.5038458695241
  out "Subtraction-10 frames average (threshold and flipped)":dbl[](graph)=[0.0, 0.0, 0.0, 0.0, 0.0, 0.0, 0.0, 0.0, 0.0, 0.0, 0.0, 0.0, 0.0, 0.0, 0.0, 0.0, 0.0, 0.0, 0.0, 0.0, 0.0, 0.0, 0.0, 0.0, 0.0, 0.0, 0.0, 0.0, 0.0, 0.0, 0.0, 0.0, 0.0, 0.0, 0.0, 0.0, 0.0, 0.0, 0.0, 0.0, 0.0, 0.0, 0.0, 0.0, 0.0, 0.0, 0.0, 0.0, 0.0, 0.0, 0.0, 0.0, 0.0, 0.0, 0.0, 0.0, 0.0, 0.0, 0.0, 0.0, 0.0, 0.0, 0.0, 0.0, 0.0, 0.0, 0.0, 0.0, 0.0, 0.0, 0.0, 0.0, 0.0, 0.0, 0.0, 0.0, 0.0, 0.0, 0.0, 0.0, 0.0, 0.0, 0.0, 0.0, 0.0, 0.0, 0.0, 0.0, 0.0, 0.0, 0.0, 0.0, 0.0, 0.0, 0.0, 0.0, 0.0, 0.0, 0.0, 0.0, 0.0, 0.0, 0.0, 0.0, 0.0, 0.0, 0.0, 0.0, 0.0, 0.0, 0.0, 0.0, 0.0, 0.0, 0.0, 0.0, 0.0, 0.0, 0.0, 0.0, 0.0, 0.0, 0.0, 0.0, 0.0, 0.0, 0.0, 0.0, 0.0, 0.0, 0.0, 0.0, 0.0, 0.0, 0.0, 0.0, 0.0, 0.0, 0.0, 0.0, 0.0, 0.0, 0.0, 0.0, 0.0, 0.0, 0.0, 0.0, 0.0, 0.0, 0.0, 0.0, 0.0, 0.0, 0.0, 0.0, 0.0, 0.0, 0.0, 0.0, 0.0, 0.0, 0.0, 0.0, 0.0, 0.0, 0.0, 0.0, 0.0, 0.0, 0.0, 0.0, 0.0, 0.0, 0.0, 0.0, 0.0, 0.0, 0.0, 0.0, 0.0, 0.0, 0.0, 0.0, 0.0, 0.0, 0.0, 0.0, 0.0, 0.0, 0.0, 0.0, 0.0, 0.0, 0.0, 0.0, 0.0, 0.0, 0.0, 0.0, 0.0, 0.0, 0.0, 0.0, 0.0, 0.0, 0.0, 0.0, 0.0, 0.0, 0.0, 0.0, 0.0, 0.0, 0.0, 0.0, 0.0, 0.0, 0.0, 0.0, 0.0, 0.0, 0.0, 0.0, 0.0, 0.0, 0.0, 0.0, 0.0, 0.0, 0.0, 0.0, 0.0, 0.0, 0.0, 0.0, 0.0, 0.0, 0.0, 0.0, 0.0, 0.0, 0.0, 0.0, 0.0, 0.0, 0.0, 0.0, 0.0, 0.0, 0.0, 0.0, 0.0, 0.0, 0.0, 0.0, 0.0, 0.0, 0.0, 0.0, 0.0, 0.0, 0.0, 0.0, 0.0, 0.0, 0.0, 0.0, 0.0, 0.0, 0.0, 0.0, 0.0, 0.0, 0.0, 0.0, 0.0, 0.0, 0.0, 0.0, 0.0, 0.0, 0.0, 0.0, 0.0, 0.0, 0.0, 0.0, 0.0, 0.0, 0.0, 0.0, 0.0, 0.0, 0.0, 0.0, 0.0, 0.0, 0.0, 0.0, 0.0, 0.0, 0.0, 0.0, 0.0, 0.0, 0.0, 0.0, 0.0, 0.0, 0.0, 0.0, 0.0, 0.0, 0.0, 0.0, 0.0, 0.0, 0.0, 0.0, 0.0, 0.0, 0.0, 0.0, 0.0, 0.0, 0.0, 0.0, 0.0, 0.0, 0.0, 0.0, 0.0, 0.0, 0.0, 0.0, 0.0, 0.0, 0.0, 0.0, 0.0, 0.0, 0.0, 0.0, 0.0, 0.0, 0.0, 0.0, 0.0, 0.0, 0.0, 0.0, 0.0, 0.0, 0.0, 0.0, 0.0, 0.0, 0.0, 0.0, 0.0, 0.0, 0.0, 0.0, 0.0, 0.0, 0.0, 0.0, 0.0, 0.0, 0.0, 0.0, 0.0, 0.0, 0.0, 0.0, 0.0, 0.0, 0.0, 0.0, 0.0, 0.0, 0.0, 0.0, 0.0, 0.0, 0.0, 0.0, 0.0, 0.0, 0.0, 0.0, 0.0, 0.0, 0.0, 0.0, 0.0, 0.0, 0.0, 0.0, 0.0, 0.0, 0.0, 0.0, 0.0, 0.0, 0.0, 0.0, 0.0, 0.0, 0.0, 0.0, 0.0, 0.0, 0.0, 0.0, 0.0, 0.0, 0.0, 0.0, 0.0, 0.0, 0.0, 0.0, 0.0, 0.0, 0.0, 0.0, 0.0, 0.0, 0.0, 0.0, 0.0, 0.0, 0.0, 0.0, 0.0, 0.0, 0.0, 0.0, 0.0, 0.0, 0.0, 0.0, 0.0, 0.0, 0.0, 0.0, 0.0, 0.0, 0.0, 0.0, 0.0, 0.0, 0.0, 0.0, 0.0, 0.0, 0.0, 0.0, 0.0, 0.0, 0.0, 0.0, 0.0, 0.0, 0.0, 0.0, 0.0, 0.0, 0.0, 0.0, 0.0, 0.0, 0.0, 0.0, 0.0, 0.0, 0.0, 0.0, 0.0, 0.0, 0.0, 0.0, 0.0, 0.0, 0.0, 0.0, 0.0, 0.0, 0.0, 0.0, 0.0, 0.0, 0.0, 0.0, 0.0, 0.0, 0.0, 0.0, 0.0, 0.0, 0.0, 0.0, 0.0, 0.0, 0.0, 0.0, 0.0, 0.0, 0.0, 0.0, 0.0, 0.0, 0.0, 0.0, 0.0, 0.0015670103505882691, 0.009835162018197504, 0.029616981315390506, 0.0625014042989501, 0.1128672492615259, 0.18893829900662376, 0.29738855173323925, 0.44223295825623055, 0.6266176323046234, 0.8530721043548897, 1.1195086267764147, 1.4210912037033385, 1.7579488476005198, 2.132581663522992, 2.5443857111810946, 2.9911684792637425, 3.468324330744002, 3.967399669097878, 4.483873119162557, 5.022939628251187, 5.593678904351159, 6.203838755444227, 6.857755021041721, 7.551353240776067, 8.273270190466423, 9.013315955611118, 9.762381248785578, 10.508042346645308, 11.240204913753823, 11.958602176812073, 12.673976795087388, 13.402935642992084, 14.154512006459548, 14.921071503776977, 15.68647722967134, 16.437586723403527, 17.168123865894394, 17.879761827917736, 18.578535061483343, 19.267315509630166, 19.94065485107036, 20.587907926490743, 21.20061134804935, 21.773362012470162, 22.303608716104222, 22.793208356915386, 23.247017737729212, 23.669613741528863, 24.062235930611784, 24.42280126710537, 24.749382026038226, 25.045450584475503, 25.318671827800443, 25.57254918261367, 25.80798889748239, 26.030394943548952, 26.24476362311442, 26.449039082604603, 26.633740599884508, 26.785680551654124, 26.895247326618097, 26.958329591603263, 26.97231793349423, 26.932711936450882, 26.83478494473758, 26.680241640654486, 26.47922779272328, 26.240185712318198, 25.96186313058943, 25.641242275096147, 25.281839996437817, 24.88936476166169, 24.465161338335747, 24.009952193974744, 23.52962875232784, 23.02966405787837, 22.50927012482069, 21.965076537470125, 21.393112719774017, 20.78836989048062, 20.14904855006249, 19.476236951774425, 18.768559616432118, 18.025284662101672, 17.251110223283675, 16.4506572222573, 15.622305852443837, 14.761166544450004, 13.865592832437217, 12.940138535050163, 11.990442677515443, 11.018400835304778, 10.026710946448254, 9.018377046715681, 7.993209335224144, 6.955237075219014, 5.918833408849362, 4.905527908146546, 3.938882350810046, 3.040910829708238, 2.2297850167548834, 1.5185773006845253, 0.9148116840918452, 0.42061396168423154, 0.033277641146948075, -0.25391101488384754, -0.45071787436917377, -0.5689777740820747, -0.6216598772948659, -0.6220350118161854, -0.5829782423007939, -0.5164229367698447, -0.4329689102945371, -0.34163679474788267, -0.24975337699672212, -0.1629479501462467, -0.08523734797621368, -0.0191768624275769, 0.033944746396776505, 0.07388585532560793, 0.10122512116673613, 0.11714092258053928, 0.12320759321881623, 0.1212157781470316, 0.1130213522923148, 0.10042482109888484, 0.08508104144793928, 0.06843747802508315, 0.05169803812773066, 0.03580877401874596, 0.021461357353519072, 0.009110155824285256, -0.0010010856369361914, -0.008806601489307852, -0.01438316394706807, -0.017914458859385547, -0.019657322877674833, -0.019911326791130717, -0.018992672289735762, -0.017212912718820476, -0.014862624556584781, -0.012199850624656991, -0.009442908173550974, -0.006767000432727104, -0.004303981359620368, -0.0021445905669832356, -0.0003424881511090148, 0.0010805334093793217, 0.0021287113054894273, 0.0028263126637286615, 0.0032118437454117035, 0.003332745205073464, 0.0032407621363534055, 0.0029880982276751784, 0.002624395387240247, 0.0021945249467137805, 0.0017371342931631014, 0.001283862999172809, 0.0008591241265219373, 0.00048033787999283864, 0.00015850447162665864, -0.00010099086962094713, -0.00029743709498482676, -0.000433803365069504, -0.0005157592291269795, -0.0005507605895506344, -0.0005472379875448193, -0.0005139099450998233, -0.0004592320798930045, -0.00039098275090484536, -0.00031597819430329114, -0.00023990442937639526, -0.00016724950178684773, -0.00010131765849671445, -4.430654083164826e-05, 2.5708563599211424e-06, 3.8936176272048425e-05, 6.508222935043747e-05, 8.180817306000358e-05, 9.026285139125543e-05, 9.18032440302056e-05, 8.787259352768435e-05, 7.990066868139865e-05, 6.922684156872292e-05, 5.7045230912518924e-05, 4.4370096602770004e-05, 3.2018939970799924e-05, 2.0610337949553413e-05, 1.0573373197966623e-05, 2.16556830155219e-06, -4.503559198638388e-06, -9.445880576292187e-06, -1.2767143033843909e-05, -1.4640296044249864e-05, -1.5280961949059467e-05, -1.4925947354422648e-05, -1.3815323628844693e-05, -1.2178288493994586e-05, -1.0222762504495106e-05, -8.128475708787543e-06, -6.0431588612096455e-06, -4.0813653543798535e-06, -2.325407828765382e-06, -8.278893798237667e-07, 3.846647960387457e-07, 1.3075216719983282e-06, 1.9531847587151984e-06, 2.346882858354879e-06, 2.5223454965963513e-06, 2.5180377119313567e-06, 2.373963016215043e-06, 2.1290875201931016e-06, 1.819391782633431e-06, 1.4765204108781223e-06, 1.1269726649244673e-06, 7.917596351974685e-07, 4.864439527247501e-07, 2.214752015170936e-07, 2.7368833971454915e-09, -1.6777242423565418e-07, -2.911914656684078e-07, -3.7103873545350995e-07, -4.1248947989521215e-07, -4.217200289414555e-07, -4.0534120772317083e-07, -3.699327881554181e-07, -3.2168264893914156e-07, -2.6612764931772895e-07, -2.0798820007495557e-07, -1.510850521629356e-07, -9.832476777581503e-08, -5.173949418667696e-08, -1.256680656270379e-08, 1.8643704948562634e-08, 4.1908975919676554e-08, 5.768621337892809e-08, 6.674996284383223e-08, 7.007863209795617e-08, 6.87547215918295e-08, 6.388130534203529e-08, 5.6515835377881136e-08, 4.762113731982407e-08, 3.80325332412121e-08, 2.8439362005429538e-08, 1.937874528207435e-08, 1.1239239047963183e-08, 4.271979974447629e-09, -1.392953978888771e-09, -5.7270363828919865e-09, -8.782424705409298e-09, -1.0671199320762074e-08]
  out "Integral of fly movement":dbl(graph)=46937.50000197561
  out "Subtraction-10 frames average (threshold and flipped) 2":dbl[](graph)=[0.0, 0.0, 0.0, 0.0, 0.0, 0.0, 0.0, 0.0, 0.0, 0.0, 0.0, 0.0, 0.0, 0.0, 0.0, 0.0, 0.0, 0.0, 0.0, 0.0, 0.0, 0.0, 0.0, 0.0, 0.0, 0.0, 0.0, 0.0, 0.0, 0.0, 0.0, 0.0, 0.0, 0.0, 0.0, 0.0, 0.0, 0.0, 0.0, 0.0, 0.0, 0.0, 0.0, 0.0, 0.0, 0.0, 0.0, 0.0, 0.0, 0.0, 0.0, 0.0, 0.0, 0.0, 0.0, 0.0, 0.0, 0.0, 0.0, 0.0, 0.0, 0.0, 0.0, 0.0, 0.0, 0.0, 0.0, 0.0, 0.0, 0.0, 0.0, 0.0, 0.0, 0.0, 0.0, 0.0, 0.0, 0.0, 0.0, 0.0, 0.0, 0.0, 0.0, 0.0, 0.0, 0.0, 0.0, 0.0, 0.0, 0.0, 0.0, 0.0, 0.0, 0.0, 0.0, 0.0, 0.0, 0.0, 0.0, 0.0, 0.0, 0.0, 0.0, 0.0, 0.0, 0.0, 0.0, 0.0, 0.0, 0.0, 0.0, 0.0, 0.0, 0.0, 0.0, 0.0, 0.0, 0.0, 0.0, 0.0, 0.0, 0.0, 0.0, 0.0, 0.0, 0.0, 0.0, 0.0, 0.0, 0.0, 0.0, 0.0, 0.0, 0.0, 0.0, 0.0, 0.0, 0.0, 0.0, 0.0, 0.0, 0.0, 0.0, 0.0, 0.0, 0.0, 0.0, 0.0, 0.0, 0.0, 0.0, 0.0, 0.0, 0.0, 0.0, 0.0, 0.0, 0.0, 0.0, 0.0, 0.0, 0.0, 0.0, 0.0, 0.0, 0.0, 0.0, 0.0, 0.0, 0.0, 0.0, 0.0, 0.0, 0.0, 0.0, 0.0, 0.0, 0.0, 0.0, 0.0, 0.0, 0.0, 0.0, 0.0, 0.0, 0.0, 0.0, 0.0, 0.0, 0.0, 0.0, 0.0, 0.0, 0.0, 0.0, 0.0, 0.0, 0.0, 0.0, 0.0, 0.0, 0.0, 0.0, 0.0, 0.0, 0.0, 0.0, 0.0, 0.0, 0.0, 0.0, 0.0, 0.0, 0.0, 0.0, 0.0, 0.0, 0.0, 0.0, 0.0, 0.0, 0.0, 0.0, 0.0, 0.0, 0.0, 0.0, 0.0, 0.0, 0.0, 0.0, 0.0, 0.0, 0.0, 0.0, 0.0, 0.0, 0.0, 0.0, 0.0, 0.0, 0.0, 0.0, 0.0, 0.0, 0.0, 0.0, 0.0, 0.0, 0.0, 0.0, 0.0, 0.0, 0.0, 0.0, 0.0, 0.0, 0.0, 0.0, 0.0, 0.0, 0.0, 0.0, 0.0, 0.0, 0.0, 0.0, 0.0, 0.0, 0.0, 0.0, 0.0, 0.0, 0.0, 0.0, 0.0, 0.0, 0.0, 0.0, 0.0, 0.0, 0.0, 0.0, 0.0, 0.0, 0.0, 0.0, 0.0, 0.0, 0.0, 0.0, 0.0, 0.0, 0.0, 0.0, 0.0, 0.0, 0.0, 0.0, 0.0, 0.0, 0.0, 0.0, 0.0, 0.0, 0.0, 0.0, 0.0, 0.0, 0.0, 0.0, 0.0, 0.0, 0.0, 0.0, 0.0, 0.0, 0.0, 0.0, 0.0, 0.0, 0.0, 0.0, 0.0, 0.0, 0.0, 0.0, 0.0, 0.0, 0.0, 0.0, 0.0, 0.0, 0.0, 0.0, 0.0, 0.0, 0.0, 0.0, 0.0, 0.0, 0.0, 0.0, 0.0, 0.0, 0.0, 0.0, 0.0, 0.0, 0.0, 0.0, 0.0, 0.0, 0.0, 0.0, 0.0, 0.0, 0.0, 0.0, 0.0, 0.0, 0.0, 0.0, 0.0, 0.0, 0.0, 0.0, 0.0, 0.0, 0.0, 0.0, 0.0, 0.0, 0.0, 0.0, 0.002507216560941266, 0.015666614324645556, 0.048414529367267235, 0.10313440140338344, 0.17806738457215382, 0.27638400615030273, 0.40850251946819616, 0.5826561862390891, 0.8008618061615357, 1.0653420537211697, 1.374836621626359, 1.7162886000050817, 2.073775278150525, 2.442047707571892, 2.8262619457227838, 3.2332631070768025, 3.6638833247839324, 4.1136951734422835, 4.579809216262396, 5.064560309861075, 5.571264949596996, 6.095727468266008, 6.62812785721717, 7.1635834482372625, 7.702333598059364, 8.240753530099408, 8.771971617054342, 9.296659141199958, 9.824764622439657, 10.366485706278588, 10.92791780350326, 11.512804570909568, 12.12125987778636, 12.746511131548859, 13.378984827940439, 14.012759197101206, 14.644809431979695, 15.274947129931881, 15.908813105263839, 16.550924294039927, 17.197230457061497, 17.843374114517147, 18.48851003277664, 19.130558547899923, 19.771000532000166, 20.417111106324278, 21.075941039014047, 21.749986513010082, 22.437472533298543, 23.13639088145387, 23.844792525523793, 24.559886291371047, 25.280428260286897, 26.009447289427165, 26.755456335369214, 27.52723984130693, 28.326338457814444, 29.147237324104637, 29.984786306320444, 30.835579270324367, 31.690676129152138, 32.536063628333835, 33.359065546718305, 34.14927245379277, 34.897299434386625, 35.59546833315736, 36.23847089177154, 36.822675376943465, 37.34857469647627, 37.822502506534164, 38.249212490939925, 38.62591571145494, 38.948660038589445, 39.22057263619253, 39.45050075826299, 39.646533528351895, 39.81284096272003, 39.95183728361499, 40.06374034836224, 40.1427461259492, 40.18177498996225, 40.17789685256884, 40.130245076296205, 40.037948478777665, 39.901557298089, 39.72642950926712, 39.519874781389866, 39.28320140062926, 39.00776666080765, 38.67973564878157, 38.290036945837116, 37.83863753465352, 37.33001742712581, 36.765885899438324, 36.14446487636626, 35.46651384981923, 34.73684375147922, 33.95978011138459, 33.137666816599136, 32.27278097572319, 31.368467369173967, 30.430622800968795, 29.46546101901217, 28.471160275386435, 27.439228633408575, 26.366710984784408, 25.257914605641524, 24.1165739819294, 22.945198165127387, 21.751653818211928, 20.548157779647365, 19.342432544257157, 18.134251221825792, 16.917539596906334, 15.683205954797899, 14.423595619519771, 13.136084554575138, 11.819644378242469, 10.473415312568882, 9.105397955106326, 7.737250162256155, 6.399218995122498, 5.123550865904613, 3.9399204295022847, 2.872536212783016, 1.9385967771303432, 1.1477941520232, 0.5025902011410339, -0.0009751299881771841, -0.3721488848055948, -0.6241720459243078, -0.7729611035089212, -0.8358633182195697, -0.8305542848186875, -0.7741198332640722, -0.6823420345204461, -0.5691912287058133, -0.4465124490780447, -0.32388507713625614, -0.2086285979186188, -0.10592441105227426, -0.019023231227144097, 0.05049088374432922, 0.10240594768529054, 0.13757918671595867, 0.15764393311998295, 0.1647399305767762, 0.16127650625935747, 0.14973423537378766, 0.13250740449472775, 0.11178684900975283, 0.08948062348416182, 0.06716844712493636, 0.046084904138771955, 0.027125903624754137, 0.010872835891032592, -0.002370883512064254, -0.01253569883065571, -0.019738394948350526, -0.024234603368385534, -0.02637399808531339, -0.02656010274857497, -0.025215945026465333, -0.022756191767973246, -0.019565894551659038, -0.01598557581877214, -0.012302090107452415, -0.008744496454637495, -0.005484066345455407, -0.0026375136774829753, -0.0002725548393658878, 0.0015850262232665468, 0.002943534901660944, 0.0038373545858983865, 0.004319251556597223, 0.004453355842469689, 0.0043090605150068175, 0.003955976995729938, 0.0034599945548559625, 0.0028804198536812667, 0.002268117395202728, 0.0016645333382224623, 0.0011014617804312613, 0.000601402300797686, 0.00017835796526951238, -0.00016106825319188016, -0.0004164059403924115, -0.0005919872933464482, -0.0006956429012188081, -0.0007374904600494944, -0.0007288635657819155, -0.0006814094723785729, -0.0006063688685042619, -0.0005140376658841887, -0.00041340062147396427, -0.00031191926326144077, -0.00021545184324920505, -0.00012828058973076917, -5.3221003759286174e-05, 8.211054453049759e-06, 5.5596608505313514e-05, 8.939435854054577e-05, 0.00011072091226774912, 0.00012114285994809677, 0.00012248969322173299, 0.00011669341219954827, 0.00010565788111035373, 9.115865344046231e-05, 7.477212528641314e-05, 5.783148909708864e-05, 4.14060213844254e-05, 2.6299700706527097e-05, 1.3064957532522651e-05, 2.0274405917046533e-06, -6.682021068039328e-06, -1.3091638109814746e-05, -1.7351907059344366e-05, -1.970015197328063e-05, -2.042805665804812e-05, -1.985334042705061e-05, -1.829624379725893e-05, -1.6061074324428943e-05, -1.3422724650516662e-05, -1.0617816413894041e-05, -7.839941765416986e-06, -5.238362082905027e-06, -2.9194719213185884e-06, -9.503347541570801e-07, 6.363653394380072e-07, 1.8365459530496355e-06, 2.668628190405467e-06, 3.1675297327907646e-06, 3.3790646530444027e-06, 3.354972973859355e-06, 3.1487184509922794e-06, 2.812119499958635e-06, 2.3928172657262186e-06, 1.9325371668130534e-06, 1.4660655610317025e-06, 1.0208405463435474e-06, 6.170439263936521e-07, 2.680783503956665e-07, -1.8682232820305408e-08, -2.409711989004527e-07, -4.0062624662619165e-07, -5.025788780146264e-07, -5.538944954686978e-07, -5.629055640556186e-07, -5.384656971340867e-07, -4.893396039238219e-07, -4.237329407920402e-07, -3.4895739556821744e-07, -2.7121980983432905e-07, -1.9551968850687653e-07, -1.2563685055518215e-07, -6.418997299279064e-08, -1.274707579640505e-08, 2.8029715293981596e-08, 5.8220799922373366e-08, 7.84803734373567e-08, 8.987295153535555e-08, 9.372312281232547e-08, 9.14839999227371e-08, 8.462758503413809e-08, 7.455832932507073e-08, 6.254958701913161e-08, 4.970145124067221e-08, 3.691759865297685e-08, 2.4898232423841318e-08, 1.4145957166592797e-08, 4.981397159258544e-09, -2.434470058871928e-09, -8.073998170208512e-09, -1.2014926023003749e-08, -1.441272344669942e-08, -1.547470982627999e-08, -1.5436999700990535e-08, -1.4544938476142128e-08, -1.3037349626558023e-08, -1.1134630681566902e-08, -9.03051194543155e-09, -6.887128367119495e-09, -4.832947142684552e-09, -2.9630352161644768e-09, -1.3411341758993554e-09, -3.026819906756002e-12, 1.0392784488925986e-09, 1.792960134158715e-09, 2.2797385935177352e-09, 2.5314457416114777e-09, 2.5860095935717633e-09, 2.4839862944067344e-09, 2.265712344314631e-09, 1.969098988006786e-09, 1.6280499899374264e-09, 1.2714533330667787e-09, 9.226762456483308e-10, 5.994804469677418e-10, 3.142694017538793e-10, 7.45803296982467e-11, -1.1626066223867908e-10, -2.5839301715849153e-10, -3.5464740271049003e-10, -4.0979225763171095e-10, -4.2983870024450915e-10, -4.214297350151918e-10, -3.913292455903789e-10, -3.460172603624e-10, -2.9139060298004885e-10, -2.3256234713666333e-10, -1.7374942887500608e-10, -1.182351979115691e-10, -6.839242529119728e-11, -2.5752109474012255e-11, 8.89589434625133e-12, 3.538308419973726e-11, 5.40342930970579e-11, 6.554041681256562e-11, 7.083883525270828e-11, 7.100650830828549e-11, 6.716891707229812e-11, 6.042643443548774e-11, 5.179838467411166e-11, 4.218400567728285e-11, 3.233875679286564e-11, 2.28639020776352e-11, 1.4207014748837311e-11, 6.670959024058489e-12, 4.2897231841655177e-13, -4.456344381456035e-12, -8.0120536737751e-12, -1.0333536984810293e-11, -1.1564053006380647e-11, -1.1876141923834467e-11, -1.1455506389740646e-11, -1.0487722227573808e-11, -9.147895635722496e-12, -7.593193169851863e-12, -5.9580265436031064e-12, -4.351574133697137e-12, -2.857260851987012e-12, -1.5337922873835503e-12, -4.1734154148082527e-13, 4.754884130156259e-13, 1.144263936714131e-12, 1.601168519613736e-12, 1.8675311721543142e-12, 1.9706115945405574e-12, 1.940764988302127e-12, 1.8090609820145927e-12, 1.6053892928910144e-12, 1.357050329386041e-12, 1.087802236170644e-12, 8.173166782054621e-13, 5.60983369697872e-13, 3.2999713413385193e-13, 1.316601380104397e-13, -3.016518548300851e-14, -1.5451116491552708e-13, -2.4271868651056814e-13, -2.9785163740987455e-13, -3.241445767776164e-13, -3.2650715192975674e-13, -3.10100403811924e-13, -2.799927389151506e-13, -2.408971723970767e-13, -1.9698655040656087e-13, -1.5177982991170486e-13, -1.0809005429054997e-13, -6.802328578500155e-14, -3.301728350886168e-14, -3.908974322425524e-15, 1.8979422608282268e-14, 3.5744556555249506e-14, 4.6803895982623886e-14, 5.280143758356358e-14, 5.4521611740523173e-14, 5.281438283838379e-14, 4.8533254026853485e-14, 4.248678672771646e-14, 3.5403354925950423e-14, 2.790817658541066e-14, 2.0511190247658236e-14, 1.3604055518789669e-14, 7.464426990592305e-15, 2.265653963981411e-15, -1.9098362054412302e-15, -5.055033831300829e-15, -7.222057262756574e-15, -8.506161944938648e-15, -9.030875755245517e-15, -8.934842205765206e-15, -8.360729018605128e-15]
  out "Fly real-time location 2":dbl(graph)=449.3915049700411
  out "max index(es) of difference 2":i32=449
  out "slope/fly moving speed 2":dbl(graph)=6.524815642372175
  out "s? t:f":dbl=1.0
  out "Laser ON/OFF? 2":i16(graph)=1
  out "Iteration Duration":i64=50
  out "sum":dbl
  in  "Date":string="2015Aug1"
  in  "Fly #":i32=331
  in  "Filename Code":string="E1"
  in  "LED High Period (ticks)":u32=1520
  in  "Apply":bool=TRUE
  in  "Output Enable":bool=TRUE
  in  "LED High Period (ticks) 2":u32=615
  in  "Apply 2":bool=TRUE
  in  "Output Enable 2":bool=TRUE
  out "FIFO Timed Out?":bool
  out "FIFO Timed Out? 2":bool
  in  "Double number of pixels to take per frame":u16=1536
  in  "Half-clocks between frames/Trigger frequency (us)":u16=1600
  in  "Half-clock time/FPGA loop timer(us)":u32=16
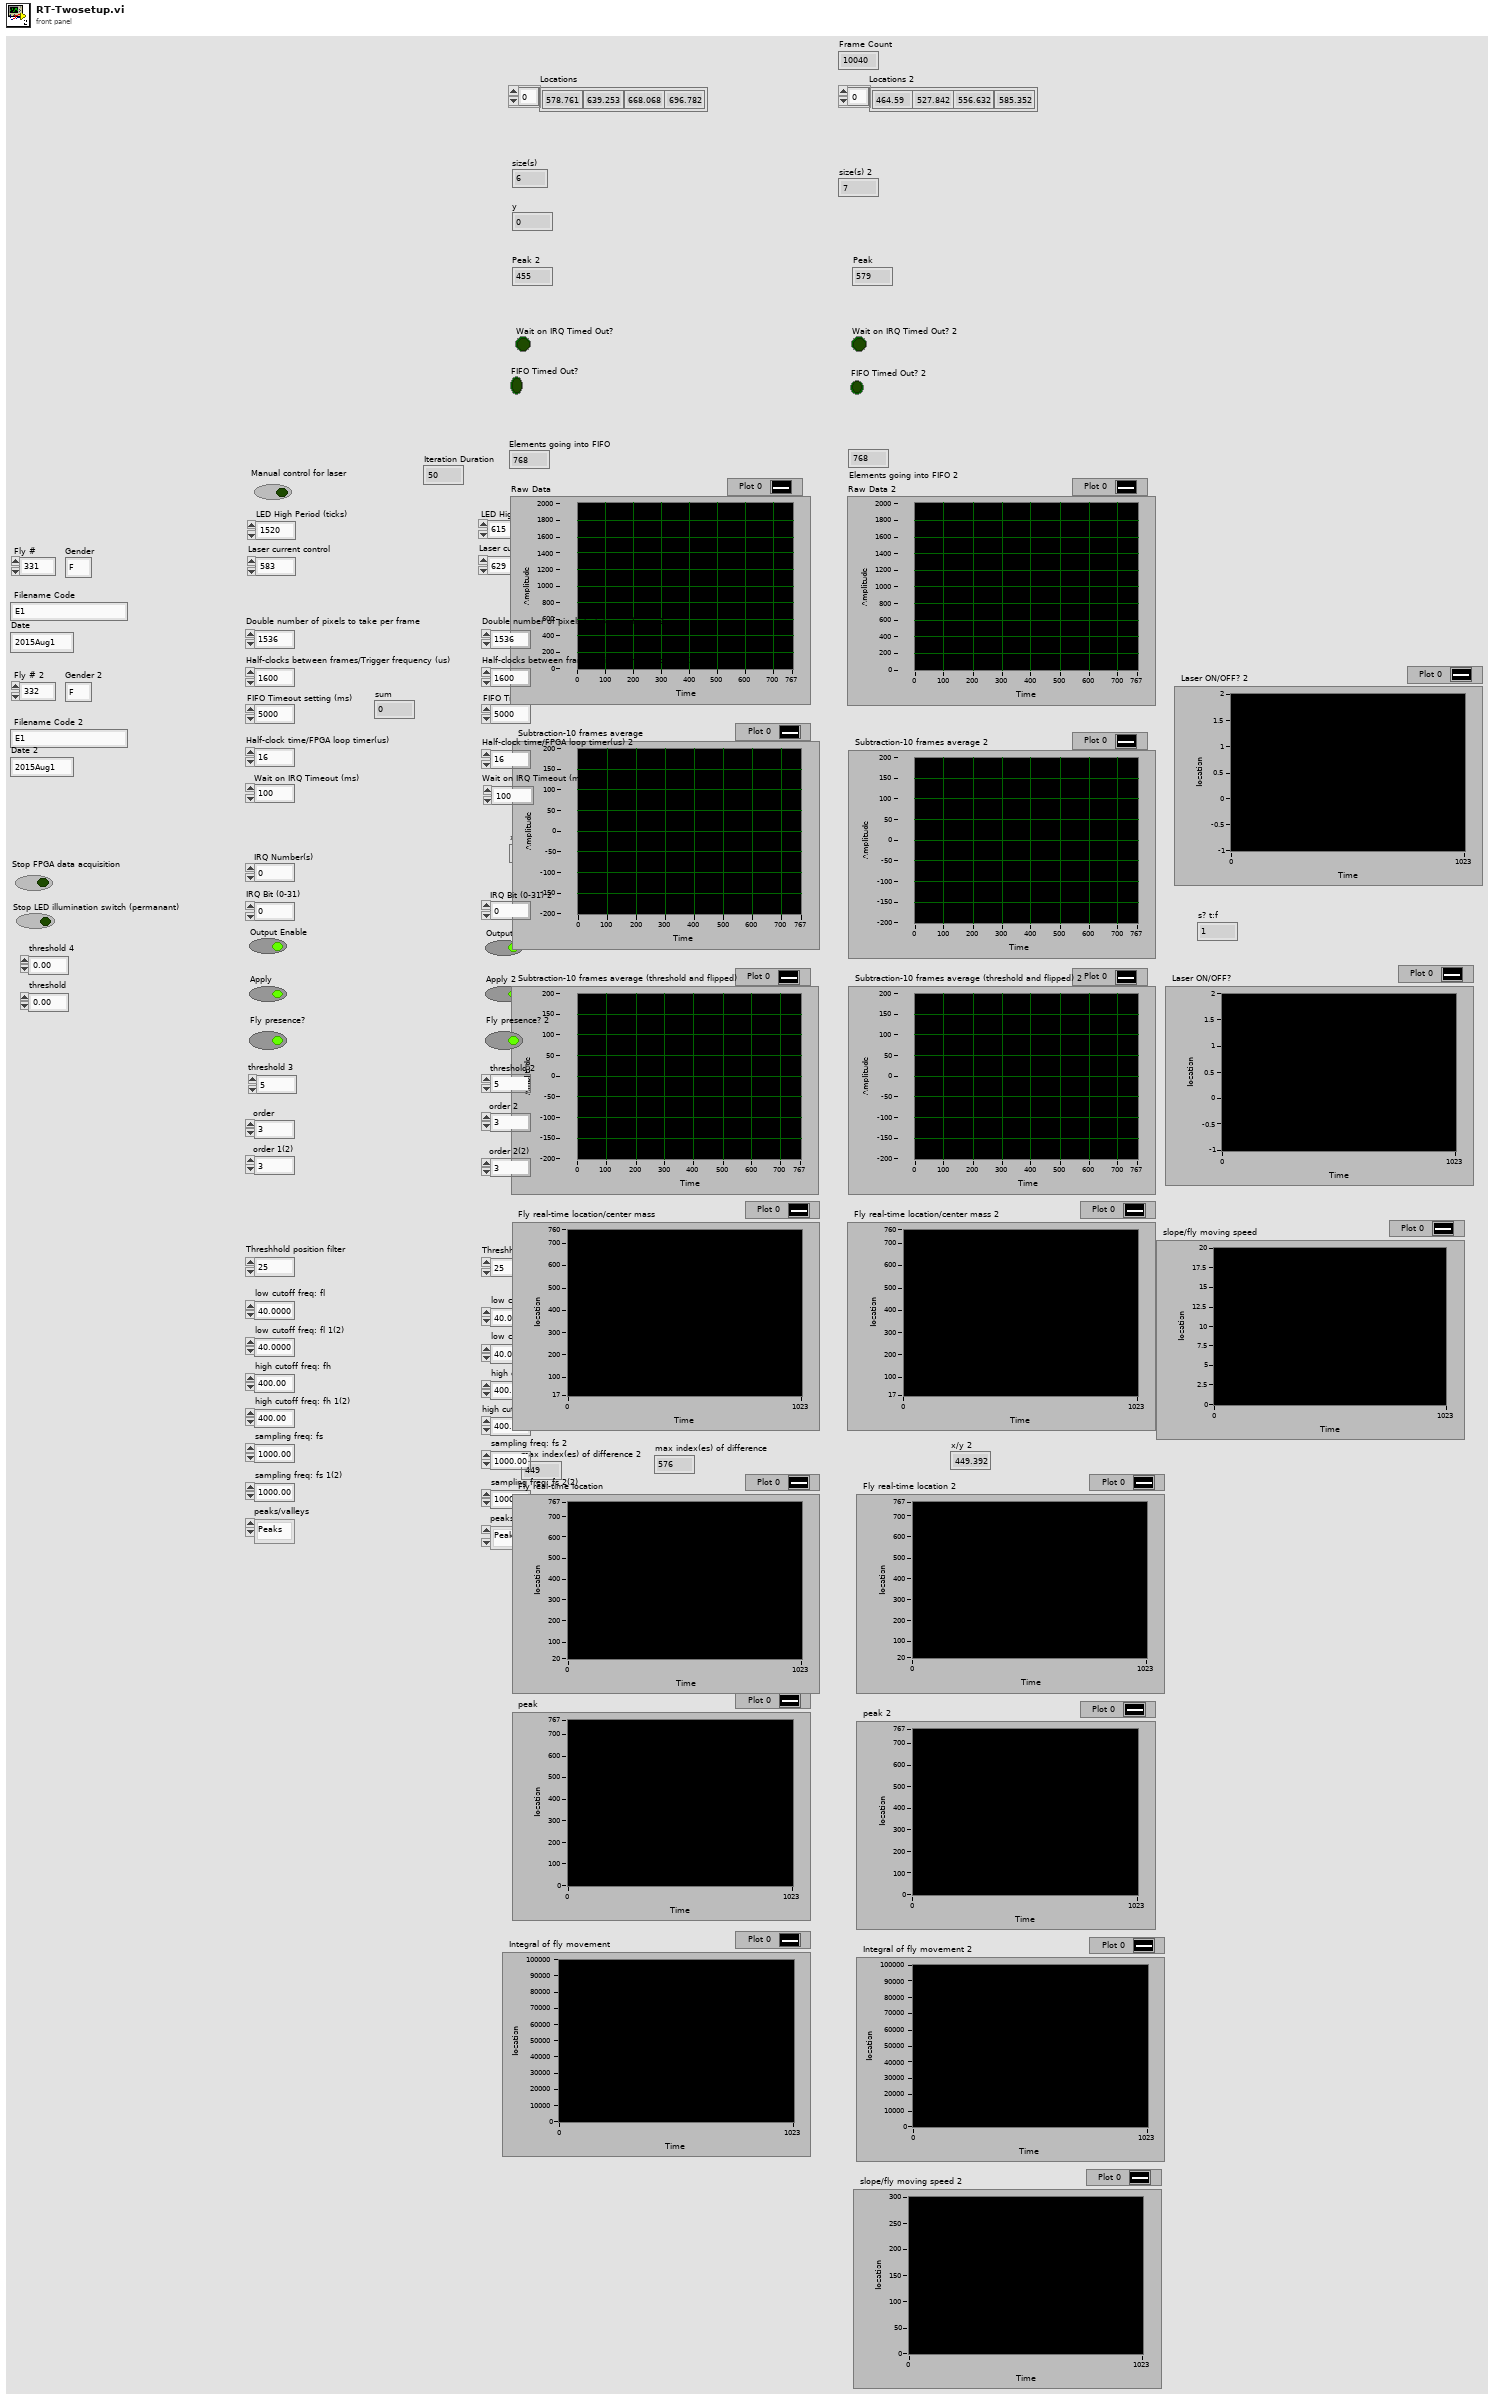
[diagram p1: front panel]
types:
  T1 = enum16{"open", "open or create", "create or replace", "create", "open (read-only)"}
  T2 = typedef "XDNodeRunTimeDep.lvlib/timing_clust.ctl" = cluster{"Expected End [f-1]":u64, "Actual End [f-1]":u64, "Finished Late? [f-1]":bool, "Expected End [i-1]":u64, "Actual End [i-1]":u64, "Finished Late? [i-1]":bool, "Expected Start [i]":u64, "Actual Start [i]":u64, "Expected Start [f]":u64, "Actual Start [f]":u64, "Source Name":string, "Structure Name":string, "Period":i64, "Deadline":i64, "Offset":i64, "Start":i64, "Priority":i32, "Timeout":i32, "Mode":T3, "Wakeup Reason":T4, "Error":errorcluster, "Source Type":string, "Secondary Source Type":string, "Global End Time":u64, "Global Start Time":u64, "Frame Duration":u64, "Iteration Duration":u64, "Assigned CPU":i32, "I/O Scan Engine Mode":u32}
  T3 = typedef "XDNodeRunTimeDep.lvlib/nitl_modes.ctl" = enum32{"No Change", "Process missed periods, maintain original phase", "Discard missed periods, maintain original phase", "Process missed periods, ignore original phase", "Discard missed periods, ignore original phase"}
  T4 = typedef "XDNodeRunTimeDep.lvlib/wakeup.ctl" = enum32{"Normal", "Aborted", "Asynchronous wakeup", "Timing source error", "Timed loop error", "Timeout"}
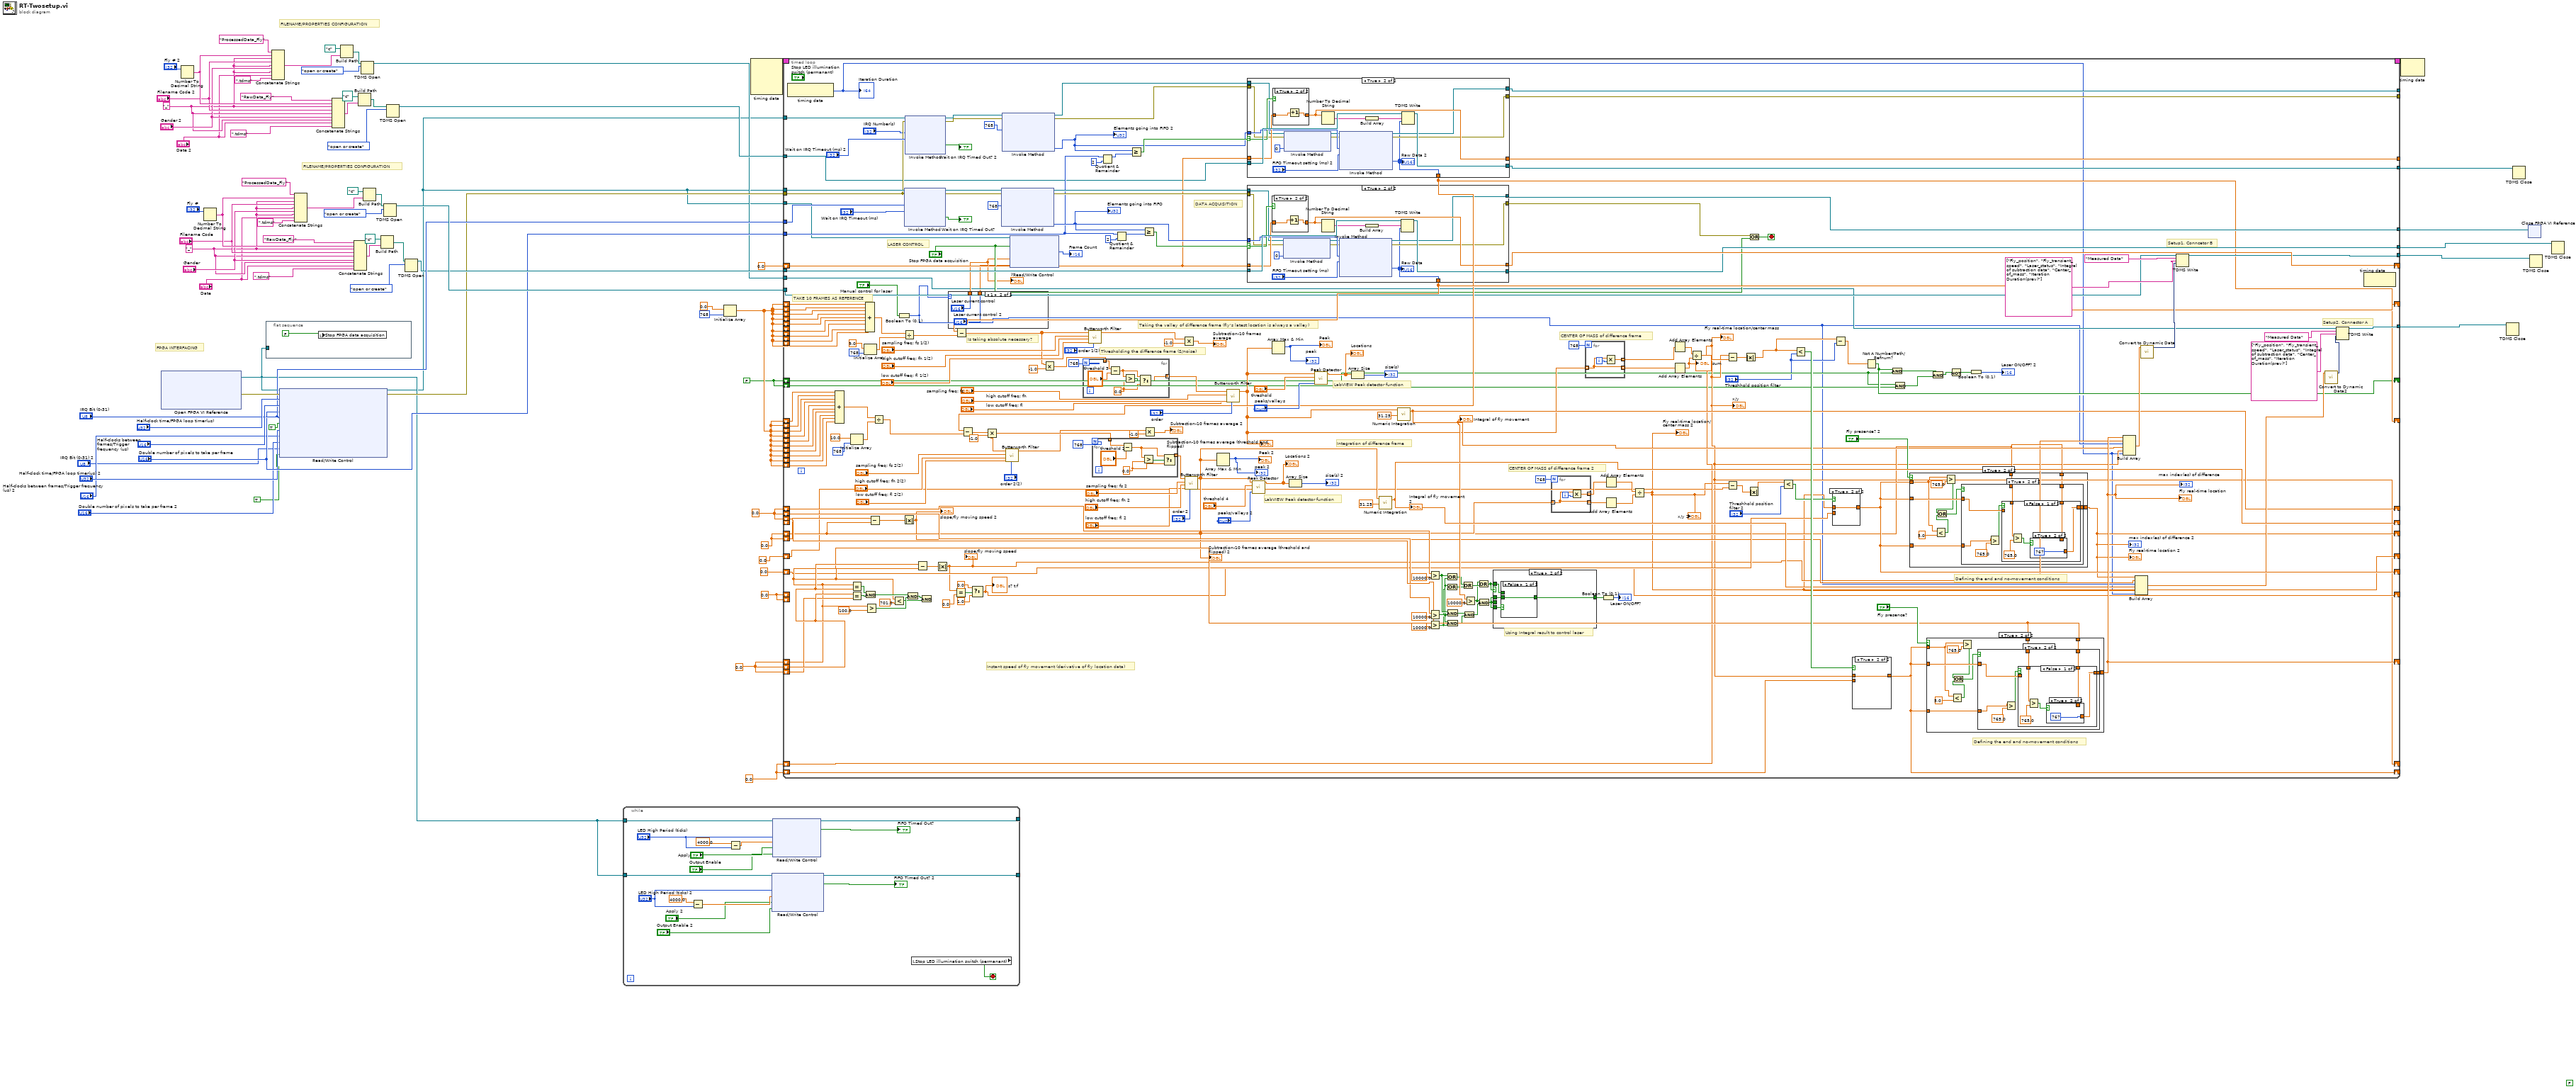
[diagram p0: block diagram]
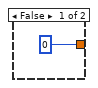
[diagram p5: hidden frame]
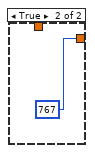
[diagram p8: hidden frame]
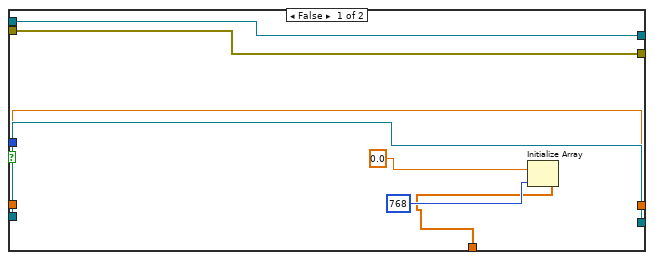
[diagram p10: hidden frame]
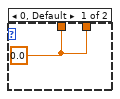
[diagram p12: hidden frame]
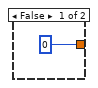
[diagram p13: hidden frame]
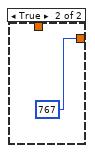
[diagram p16: hidden frame]
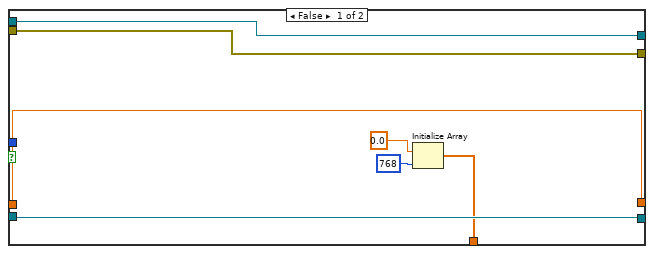
[diagram p18: hidden frame]
diagram:
  w2 = FALSE
  w3 = 0.0 ("y")
  w5 = 0.0 ("y")
  w14 = "_" ("string")
  w54 = 0.0 ("y")
  w55 = 0.0 ("y")
  (unwired) FALSE
  w56 = 0.0
  w45 = "_" ("string")
  # "FILENAME/PROPERTIES CONFIGURATION"
  # "FILENAME/PROPERTIES CONFIGURATION"
  # "FPGA INTERFACING"
  n1 = xnode "Open FPGA VI Reference"() -> ("FPGA VI Reference Out"=w30:refnum<k20>, "error out"=w61:errorcluster)  [unwired: 2 in]
  n2 = Number To Decimal String(number="Fly # 2") -> (decimal integer string=w18:string)  [unwired: 1 in]
  n3 = Number To Decimal String(number="Fly #") -> (decimal integer string=w49:string)  [unwired: 1 in]
  n4 = flat-sequence {
    tunnel: w30 -> [_]
    frame #0 {
      n5 = local write "Stop FPGA data acquisition"(FALSE ("Stop")) -> ()
    }
  }
  n6 = Concatenate Strings("ProcessedData_Fly" ("string"), w18, w14, "Filename Code 2", w14, "Gender 2", w14, "Date 2", ".tdms" ("string")) -> (w25:string)
  n7 = xnode "Read/Write Control"("FPGA VI Reference In"=w30, "error in"=w61, "Half-clock time"="Half-clock time/FPGA loop timer(us)", "Half-clocks between frames"="Half-clocks between frames/Trigger frequency (us)", "double number of samples to take per frame"="Double number of pixels to take per frame", "IRQ Bit (0-31)"="IRQ Bit (0-31)", "Wait Until IRQ Cleared?"=TRUE, "Half-clock time 2"="Half-clock time/FPGA loop timer(us) 2", "Half-clocks between frames 2"="Half-clocks between frames/Trigger frequency (us) 2", "double number of samples to take per frame 2"="Double number of pixels to take per frame 2", "IRQ Bit (0-31) 2"="IRQ Bit (0-31) 2", "Wait Until IRQ Cleared? 2"=TRUE ("Wait Until IRQ Cleared?")) -> ("FPGA VI Reference Out"=w1:refnum<k20>, "error out"=w38:errorcluster)
  n8 = Concatenate Strings("ProcessedData_Fly" ("string"), w49, w45, "Filename Code", w45, "Gender", w45, "Date", ".tdms" ("string")) -> (w66:string)
  n9 = Concatenate Strings("RawData_Fly" ("string"), w18, w14, "Filename Code 2", w14, "Gender 2", w14, "Date 2", ".tdms" ("string")) -> (w20:string)
  n10 = Build Path(base path=path "c:/", name or relative path=w25) -> (appended path=w24:path)
  n11 = Concatenate Strings("RawData_Fly" ("string"), w49, w45, "Filename Code", w45, "Gender", w45, "Date", ".tdms" ("string")) -> (w59:string)
  n12 = Build Path(base path=path "c:/", name or relative path=w20) -> (appended path=w11:path)
  n13 = TDMS Open(10:T1."open or create" ("operation (0:open)"), 11:w24) -> (3:w8:refnum<k34>)  [unwired: 5 in, 1 out]
  n14 = Build Path(base path=path "c:/", name or relative path=w66) -> (appended path=w65:path)
  n15 = Build Path(base path=path "c:/", name or relative path=w59) -> (appended path=w70:path)
  n16 = TDMS Open(10:T1."open or create" ("operation (0:open)"), 11:w65) -> (3:w64:refnum<k34>)  [unwired: 5 in, 1 out]
  n17 = TDMS Open(10:T1."open or create" ("operation (0:open)"), 11:w11) -> (3:w10:refnum<k34>)  [unwired: 5 in, 1 out]
  n18 = TDMS Open(10:T1."open or create" ("operation (0:open)"), 11:w70) -> (3:w39:refnum<k34>)  [unwired: 5 in, 1 out]
  n19 = while {
    tunnel: w30 -> [w91]
    tunnel: [w90] -> _
    tunnel: w30 -> [w83]
    tunnel: [w82] -> _
    stop <- w89 stop-if-true
    n20 = Subtract(x=4000.0, y="LED High Period (ticks) 2") -> (x-y=w79:dbl)
    n21 = Subtract(x=4000.0, y="LED High Period (ticks)") -> (x-y=w87:dbl)
    n22 = xnode "Read/Write Control"("FPGA VI Reference In"=w83, "High Period (ticks) 2"="LED High Period (ticks) 2", "Low Period (ticks) 2"=w79, "Apply 2"="Apply 2", "Output Enable 2"="Output Enable 2") -> ("FPGA VI Reference Out"=w82:refnum<k20>, "Timed Out? 2"=→"FIFO Timed Out? 2":bool)  [unwired: 1 in, 1 out]
    n23 = xnode "Read/Write Control"("FPGA VI Reference In"=w91, "High Period (ticks)"="LED High Period (ticks)", "Low Period (ticks)"=w87, "Apply"="Apply", "Output Enable"="Output Enable") -> ("FPGA VI Reference Out"=w90:refnum<k20>, "Timed Out?"=→"FIFO Timed Out?":bool)  [unwired: 1 in, 1 out]
    n24 = local read "Stop LED illumination switch (permanant)"() -> (w89:bool)
  }
  n25 = Initialize Array(0.0 ("element"), 768 ("dimension size")) -> (w29:dbl[])
  n26 = node-c288 ("Input Node")() -> (w73:T2)  [unwired: 4 in]
  n27 = timed-loop {
    tunnel: "Double number of pixels to take per frame" -> [w235]
    tunnel: w1 -> [w243]
    tunnel: [w310] -> w58
    tunnel: w38 -> [w242]
    tunnel: w39 -> [w230]
    tunnel: [w295] -> w51
    tunnel: "IRQ Bit (0-31)" -> [w241]
    tunnel: w64 -> [w140]
    tunnel: [w261] -> w57
    shift-right: [w305] -> _
    shift-left: 0.0 -> [w231]
    shift-right: [w108] -> _
    shift-left: w56 -> [w132]
    shift-right: [w301] -> _
    shift-left: w56 -> [w189]
    timing: w73 -> [_]
    timing-out: [_] -> w72
    shift-right: [w205] -> _
    shift-left: w29 -> [w222]
    shift-left: w29 -> [w221]
    shift-left: w29 -> [w220]
    shift-left: w29 -> [w219]
    shift-left: w29 -> [w218]
    shift-left: w29 -> [w217]
    shift-left: w29 -> [w216]
    shift-left: w29 -> [w215]
    shift-left: w29 -> [w214]
    shift-right: [w300] -> _
    shift-left: w55 -> [w186]
    shift-left: w55 -> [w286]
    shift-left: w55 -> [w285]
    shift-right: [w153] -> _
    shift-left: w54 -> [w275]
    shift-left: w54 -> [w211]
    shift-left: w54 -> [w271]
    tunnel: [w229] -> _
    tunnel: [w228] -> _
    tunnel: [w227] -> _
    tunnel: [w226] -> w9
    shift-right: [w194] -> _
    shift-left: _ -> [_]
    shift-right: [w187] -> _
    shift-left: 0.0 ("y") -> [w138]
    shift-right: [w169] -> _
    shift-left: w29 -> [w184]
    shift-left: w29 -> [w183]
    shift-left: w29 -> [w182]
    shift-left: w29 -> [w181]
    shift-left: w29 -> [w180]
    shift-left: w29 -> [w179]
    shift-left: w29 -> [w178]
    shift-left: w29 -> [w177]
    shift-left: w29 -> [w176]
    shift-left: w29 -> [w175]
    tunnel: [w171] -> w7
    tunnel: w10 -> [w141]
    tunnel: w8 -> [w139]
    shift-right: [w137] -> _
    shift-left: w5 -> [w135]
    shift-left: w5 -> [w136]
    shift-right: [w109] -> _
    shift-left: 0.0 ("y") -> [w110]
    shift-right: [w125] -> _
    shift-left: w3 -> [_]
    shift-left: w3 -> [_]
    shift-right: [w107] -> _
    shift-left: w2 -> [w106]
    shift-left: w2 -> [w105]
    tunnel: w1 -> [w93]
    tunnel: w1 -> [w92]
    stop <- w309 stop-if-true
    # "Setup2, Connector A"
    # "Setup1, Conncetor B"
    # "Defining the end and no-movement conditions"
    # "CENTER OF MASS of difference frame 2"
    # "LabVIEW Peak detector function"
    # "Instant speed of fly movement (derivative of fly location data)"
    # "Defining the end and no-movement conditions"
    # "CENTER OF MASS of difference frame"
    # "Using Integral result to control laser"
    # "Integration of difference frame"
    # "LabVIEW Peak detector function"
    # "Thresholding the difference frame (S/noise)"
    # "Taking the valley of difference frame (fly's latest location is always a valley)"
    # "Is taking absolute necessary?"
    # "TAKE 10 FRAMES AS REFERENCE"
    # "LASER CONTROL"
    # "DATA ACQUISITION"
    n28 = node-c288() -> (w94:i64)  [unwired: 1 in]
    "Iteration Duration" <- w94
    n29 = Compound Arithmetic op=ADD(w184, w183, w182, w181, w180, w179, w178, w177, w176, w175) -> (w213:dbl[])
    n30 = Initialize Array(10.0 ("element"), 768 ("dimension size")) -> (w212:dbl[])
    n31 = Equal?(x=w186, y=w286) -> (x = y?=w284:bool)
    n32 = Equal?(x=w286, y=w285) -> (x = y?=w283:bool)
    n33 = Initialize Array(9.0 ("element"), 768 ("dimension size")) -> (w258:dbl[])
    n34 = And(x=w284, y=w283) -> (x .and. y?=w280:bool)
    n35 = Compound Arithmetic op=ADD(w222, w221, w220, w219, w218, w217, w216, w215, w214) -> (w259:dbl[])
    n36 = Greater?(x=w186, y=100.0) -> (0:w281:bool)
    n37 = Subtract(x=w136, y=w135) -> (x-y=w134:dbl)
    n38 = Divide(x=w213, y=w212) -> (x/y=w170:dbl[])
    n39 = Less?(x=w186, y=701.0) -> (x < y?=w277:bool)
    n40 = Boolean To (0,1)(Boolean="Manual control for laser") -> (0, 1=w96:i16)
    n41 = Absolute Value(x=w134) -> (abs(x)=w133:dbl)
    "slope/fly moving speed 2" <- w133
    n42 = Divide(x=w259, y=w258) -> (x/y=w260:dbl[])
    n43 = xnode "Invoke Method"("FPGA VI Reference In"=w243, "error in"=w242, "IRQ Number(s)"=w241, "Timeout (ms)"="Wait on IRQ Timeout (ms)") -> ("FPGA VI Reference Out"=w265:refnum<k20>, "error out"=w263:errorcluster, "Timed Out"=→"Wait on IRQ Timed Out?":bool)  [unwired: 1 out]
    n44 = xnode "Invoke Method"("FPGA VI Reference In"=w93, "error in"=w242, "IRQ Number(s)"="IRQ Number(s)", "Timeout (ms)"="Wait on IRQ Timeout (ms) 2") -> ("FPGA VI Reference Out"=w239:refnum<k20>, "error out"=w240:errorcluster, "Timed Out"=→"Wait on IRQ Timed Out? 2":bool)  [unwired: 1 out]
    n45 = And(x=w280, y=w281) -> (x .and. y?=w279:bool)
    n46 = Subtract(x=w286, y=w186) -> (x-y=w294:dbl)
    n47 = And(x=w279, y=w277) -> ()  [unwired: 1 out]
    n48 = Absolute Value(x=w294) -> (abs(x)=w131:dbl)
    "slope/fly moving speed" <- w131
    n49 = case shown="1" w96 {
      tunnel: [w388 "Laser current control"] -> w143
      tunnel: [w388 "Laser current control 2"] -> w95
      frame 0, Default {
        w388 = 0.0 ("y")
      }
      frame 1 {
      }
    }
    "y" <- w143
    n50 = Equal?(x=w131, y=0.0) -> (x = y?=w129:bool)
    n51 = Select(t=0.0, s=w129, f=1.0) -> (s? t:f=w125:dbl)
    "s? t:f" <- w125
    n52 = xnode "Invoke Method"("FPGA VI Reference In"=w265, "error in"=w263, "Number of Elements"=u32 768) -> ("FPGA VI Reference Out"=w264:refnum<k20>, "Elements Remaining"=w262:u32)  [unwired: 1 in, 2 out]
    "Elements going into FIFO" <- w262
    n53 = xnode "Invoke Method"("FPGA VI Reference In"=w239, "error in"=w240, "Number of Elements"=u32 768) -> ("FPGA VI Reference Out"=w233:refnum<k20>, "error out"=w232:errorcluster, "Elements Remaining"=w166:u32)  [unwired: 1 in, 1 out]
    "Elements going into FIFO 2" <- w166
    n54 = xnode "Read/Write Control"("FPGA VI Reference In"=w92, "FPGA Stop"="Stop FPGA data acquisition", "ConnectorB/AO0"=w143, "ConnectorA/AO0 2"=w95) -> ("Frame Count"=→"Frame Count":i16)  [unwired: 1 in, 2 out]
    n55 = Quotient & Remainder(x=w235, y=u16 2) -> (x-y*floor(x/y)=w236:u16)  [unwired: 1 out]
    n56 = Quotient & Remainder(x=w235, y=u16 2) -> (x-y*floor(x/y)=w308:u16)  [unwired: 1 out]
    n57 = Greater Or Equal?(x=w166, y=w236) -> (x >= y?=w234:bool)
    n58 = Greater Or Equal?(x=w262, y=w308) -> (x >= y?=w306:bool)
    n59 = case shown="True" w306 {
      selector: w306 -> [_ w453]
      tunnel: [w437 w448] -> w310
      tunnel: w230 -> [w439 w455]
      tunnel: [w439 w454] -> w261
      tunnel: w263 -> [w438 w445]
      tunnel: [w438 w447] -> w304
      tunnel: w264 -> [w437 w446]
      tunnel: w231 -> [w434 w452]
      tunnel: [w434 w451] -> w305
      tunnel: w262 -> [_ w449]
      tunnel: [w433 w440] -> w205
      frame False {
        n60 = Initialize Array(0.0 ("element"), 768 ("dimension size")) -> (w433:dbl[])
      }
      frame True {
        n61 = case shown="True" w453 {
          tunnel: w452 -> [w457 w459]
          tunnel: [w457 w458] -> w451
          frame False {
          }
          frame True {
            n62 = Increment(x=w459) -> (x+1=w458:dbl)
          }
        }
        n63 = xnode "Invoke Method"("FPGA VI Reference In"=w446, "error in"=w445, "IRQ Number(s)"=u32 0 ("Number of Elements")) -> ("FPGA VI Reference Out"=w443:refnum<k20>, "error out"=w442:errorcluster)
        n64 = Number To Decimal String(number=w451) -> (decimal integer string=w450:string)  [unwired: 1 in]
        n65 = xnode "Invoke Method"("FPGA VI Reference In"=w443, "error in"=w442, "Number of Elements"=w449, "Timeout (ms)"="FIFO Timeout setting (ms)") -> ("FPGA VI Reference Out"=w448:refnum<k20>, "error out"=w447:errorcluster, "Data"=w440:u16[])  [unwired: 1 out]
        "Raw Data" <- w440
        n66 = Build Array(w450) -> (w441:string[])
        n67 = TDMS Write(0:w455, 7:w441, 9:w440) -> (4:w454:refnum<k34>)  [unwired: 3 in, 3 out]
      }
    }
    n68 = Subtract(x=w205, y=w260) -> (x-y=w248:dbl[])
    n69 = Multiply(x=w248, y=-1.0) -> (x*y=w246:dbl[])
    n70 = for {
      N: 768 -> [_]
      tunnel: w246 -> [w399] mode=indexing
      tunnel: [w395] -> w253 mode=indexing
      w396 = 0.0 ("y")
      n71 = Subtract(x=w399, y="threshold 3") -> (x-y=w397:dbl)
      n72 = Greater?(x=w397, y=w396) -> (0:w398:bool)
      n73 = Select(t=w397, s=w398, f=w396) -> (s? t:f=w395:dbl)
    }
    n74 = call-poly <vilib>:"Butterworth Filter.vi"("order"="order 1(2)", "low cutoff freq: fl"="low cutoff freq: fl 1(2)", "high cutoff freq: fh"="high cutoff freq: fh 1(2)", "sampling freq: fs"="sampling freq: fs 1(2)", "X"=w248) -> ("Filtered X"=w269:dbl[])  [unwired: 3 in, 1 out]
    n75 = Multiply(x=w269, y=-1.0) -> (x*y=→"Subtraction-10 frames average":dbl[])
    n76 = call-poly <vilib>:"Butterworth Filter.vi"("order"="order", "low cutoff freq: fl"="low cutoff freq: fl", "high cutoff freq: fh"="high cutoff freq: fh", "sampling freq: fs"="sampling freq: fs", "X"=w253) -> ("Filtered X"=w142:dbl[])  [unwired: 3 in, 1 out]
    "Subtraction-10 frames average (threshold and flipped)" <- w142
    n77 = case shown="True" w234 {
      selector: w234 -> [_ w381]
      tunnel: [w365 w376] -> w229
      tunnel: w141 -> [w367 w383]
      tunnel: [w367 w382] -> w226
      tunnel: w232 -> [w366 w373]
      tunnel: [w366 w375] -> w228
      tunnel: w233 -> [w365 w374]
      tunnel: w231 -> [w362 w380]
      tunnel: [w362 w379] -> w227
      tunnel: w166 -> [_ w377]
      tunnel: [w361 w368] -> w169
      frame False {
        n78 = Initialize Array(0.0 ("element"), 768 ("dimension size")) -> (w361:dbl[])
      }
      frame True {
        n79 = case shown="True" w381 {
          tunnel: w380 -> [w385 w387]
          tunnel: [w385 w386] -> w379
          frame False {
          }
          frame True {
            n80 = Increment(x=w387) -> (x+1=w386:dbl)
          }
        }
        n81 = xnode "Invoke Method"("FPGA VI Reference In"=w374, "error in"=w373, "IRQ Number(s)"=u32 0 ("Number of Elements")) -> ("FPGA VI Reference Out"=w371:refnum<k20>, "error out"=w370:errorcluster)
        n82 = Number To Decimal String(number=w379) -> (decimal integer string=w378:string)  [unwired: 1 in]
        n83 = xnode "Invoke Method"("FPGA VI Reference In"=w371, "error in"=w370, "Number of Elements"=w377, "Timeout (ms)"="FIFO Timeout setting (ms) 2") -> ("FPGA VI Reference Out"=w376:refnum<k20>, "error out"=w375:errorcluster, "Data"=w368:u16[])  [unwired: 1 out]
        "Raw Data 2" <- w368
        n84 = Build Array(w378) -> (w369:string[])
        n85 = TDMS Write(0:w383, 7:w369, 9:w368) -> (4:w382:refnum<k34>)  [unwired: 3 in, 3 out]
      }
    }
    n86 = Subtract(x=w169, y=w170) -> (x-y=w149:dbl[])
    n87 = Multiply(x=w149, y=-1.0) -> (x*y=w206:dbl[])
    n88 = call-poly <vilib>:"Butterworth Filter.vi"("order"="order 2(2)", "low cutoff freq: fl"="low cutoff freq: fl 2(2)", "high cutoff freq: fh"="high cutoff freq: fh 2(2)", "sampling freq: fs"="sampling freq: fs 2(2)", "X"=w149) -> ("Filtered X"=w203:dbl[])  [unwired: 3 in, 1 out]
    n89 = for {
      N: 768 -> [_]
      tunnel: [w357] -> w204 mode=indexing
      tunnel: w206 -> [w355] mode=indexing
      w358 = 0.0 ("y")
      n90 = Subtract(x=w355, y="threshold 2") -> (x-y=w359:dbl)
      n91 = Greater?(x=w359, y=w358) -> (0:w360:bool)
      n92 = Select(t=w359, s=w360, f=w358) -> (s? t:f=w357:dbl)
    }
    n93 = Multiply(x=w203, y=-1.0) -> (x*y=→"Subtraction-10 frames average 2":dbl[])
    n94 = call-poly <vilib>:"Butterworth Filter.vi"("order"="order 2", "low cutoff freq: fl"="low cutoff freq: fl 2", "high cutoff freq: fh"="high cutoff freq: fh 2", "sampling freq: fs"="sampling freq: fs 2", "X"=w204) -> ("Filtered X"=w148:dbl[])  [unwired: 3 in, 1 out]
    "Subtraction-10 frames average (threshold and flipped) 2" <- w148
    n95 = Array Max & Min(array=w148) -> (max index (indices)=→"peak 2" →"Peak 2":i32)  [unwired: 3 out]
    n96 = call <vilib>:"Peak Detector.vi"("peaks/valleys"="peaks/valleys 2", "threshold"="threshold 4", "X"=w148) -> ("Locations"=w145:dbl[])  [unwired: 4 in, 4 out]
    "Locations 2" <- w145
    n97 = Array Max & Min(array=w142) -> (max index (indices)=→"peak" →"Peak":i32)  [unwired: 3 out]
    n98 = Array Size(array=w145) -> (size(s)=→"size(s) 2":i32)
    n99 = call <vilib>:"Peak Detector.vi"("peaks/valleys"="peaks/valleys", "threshold"="threshold", "X"=w142) -> ("Locations"=w144:dbl[])  [unwired: 4 in, 4 out]
    "Locations" <- w144
    n100 = Array Size(array=w144) -> (size(s)=→"size(s)":i32)
    n101 = call-poly <vilib>:"Numeric Integration.vi"("dt"=31.25, "Input Array"=w148) -> ("result"=w194:dbl)  [unwired: 1 in, 1 out]
    "Integral of fly movement 2" <- w194
    n102 = call-poly <vilib>:"Numeric Integration.vi"("dt"=31.25, "Input Array"=w142) -> ("result"=w153:dbl)  [unwired: 1 in, 1 out]
    "Integral of fly movement" <- w153
    n103 = Greater?(x=w275, y=10000.0) -> (0:w121:bool)
    n104 = Greater?(x=w211, y=10000.0) -> (0:w120:bool)
    n105 = Greater?(x=w271, y=10000.0) -> (0:w119:bool)
    n106 = Or(x=w121, y=w120) -> (x .or. y?=w124:bool)
    n107 = Or(x=w120, y=w119) -> (x .or. y?=w123:bool)
    n108 = And(x=w121, y=w120) -> (x .and. y?=w118:bool)
    n109 = And(x=w120, y=w119) -> (x .and. y?=w117:bool)
    n110 = Or(x=w124, y=w123) -> (x .or. y?=w122:bool)
    n111 = And(x=w118, y=w117) -> (x .and. y?=w116:bool)
    n112 = Greater?(x=w153, y=10000.0) -> (0:w115:bool)
    n113 = Or(x=w115, y=w122) -> (x .or. y?=w112:bool)
    n114 = And(x=w115, y=w116) -> (x .and. y?=w111:bool)
    n115 = case shown="True" w112 {
      tunnel: w111 -> [_ w319]
      tunnel: w111 -> [_ w318]
      tunnel: [w313 w317] -> w113
      tunnel: w112 -> [_ w316]
      tunnel: w111 -> [w312 _]
      frame False {
        n116 = case shown="False" w312 {
          tunnel: [w314 w315] -> w313
          tunnel: w312 -> [w314 _]
          tunnel: w312 -> [_ w315]
          frame False {
          }
          frame True {
          }
        }
      }
      frame True {
        n117 = case shown="False" w319 {
          tunnel: [w320 w321] -> w317
          tunnel: w318 -> [w320 _]
          tunnel: w316 -> [_ w321]
          frame False {
          }
          frame True {
          }
        }
      }
    }
    n118 = for {
      N: 768 -> [_]
      tunnel: w148 -> [w352] mode=indexing
      tunnel: [w353] -> w196 mode=indexing
      tunnel: [w352] -> w195 mode=indexing
      i -> [w354]
      n119 = Multiply(x=w352, y=w354) -> (x*y=w353:dbl)
    }
    n120 = for {
      N: 768 -> [_]
      tunnel: w142 -> [w391] mode=indexing
      tunnel: [w392] -> w292 mode=indexing
      tunnel: [w391] -> w290 mode=indexing
      i -> [w393]
      n121 = Multiply(x=w391, y=w393) -> (x*y=w392:dbl)
    }
    n122 = Boolean To (0,1)(Boolean=w113) -> (0, 1=→"Laser ON/OFF?":i16)
    n123 = Add Array Elements(numeric array=w196) -> (sum=w197:dbl)
    n124 = Add Array Elements(numeric array=w195) -> (sum=w198:dbl)
    n125 = Divide(x=w197, y=w198) -> (x/y=w109:dbl)
    "Fly real-time location/center mass 2" <- w109
    "x/y 2" <- w109
    n126 = Add Array Elements(numeric array=w292) -> (sum=w254:dbl)
    n127 = Add Array Elements(numeric array=w290) -> (sum=w289:dbl)
    "sum" <- w289
    n128 = Divide(x=w254, y=w289) -> (x/y=w108:dbl)
    "Fly real-time location/center mass" <- w108
    "x/y" <- w108
    n129 = Subtract(x=w108, y=w132) -> (x-y=w303:dbl)
    n130 = Subtract(x=w109, y=w110) -> (x-y=w193:dbl)
    n131 = Absolute Value(x=w303) -> (abs(x)=w100:dbl)
    n132 = Absolute Value(x=w193) -> (abs(x)=w192:dbl)
    n133 = Or(x=w304, y="Stop FPGA data acquisition") -> (x .or. y?=w309:bool)
    n134 = Less?(x=w192, y="Threshhold position filter 2") -> (x < y?=w190:bool)
    n135 = Less?(x=w100, y="Threshhold position filter") -> (x < y?=w302:bool)
    n136 = case shown="True" w190 {
      tunnel: w109 -> [_ w351]
      tunnel: [w350 w351] -> w187
      tunnel: w138 -> [w350 _]
      frame False {
      }
      frame True {
      }
    }
    n137 = Subtract(x=w100, y="Threshhold position filter") -> (x-y=w98:dbl)
    n138 = case shown="True" w302 {
      tunnel: w108 -> [_ w432]
      tunnel: [w431 w432] -> w301
      tunnel: w189 -> [w431 _]
      frame False {
      }
      frame True {
      }
    }
    n139 = Not A Number/Path/Refnum?(number/path/refnum=w98) -> (NaN/Path/Refnum?=w107:bool)
    n140 = And(x=w107, y=w106) -> (x .and. y?=w104:bool)
    n141 = And(x=w106, y=w105) -> (x .and. y?=w103:bool)
    n142 = case shown="True" "Fly presence? 2" {
      tunnel: w187 -> [_ w333]
      tunnel: [0 w332] -> w137
      tunnel: w187 -> [_ w326]
      tunnel: w187 -> [_ w325]
      tunnel: w135 -> [_ w324]
      tunnel: w135 -> [_ w323]
      frame False {
      }
      frame True {
        n143 = Less?(x=w326, y=5.0) -> (x < y?=w329:bool)
        n144 = Greater?(x=w326, y=765.0) -> (0:w327:bool)
        n145 = Or(x=w327, y=w329) -> (x .or. y?=w331:bool)
        n146 = case shown="True" w331 {
          tunnel: w333 -> [w334 w340]
          tunnel: [w334 w341] -> w332
          tunnel: w325 -> [_ w335]
          tunnel: w324 -> [_ w338]
          tunnel: w323 -> [_ w336]
          frame False {
          }
          frame True {
            n147 = Greater?(x=w335, y=765.0) -> (0:w337:bool)
            n148 = case shown="False" w337 {
              tunnel: [w344 767] -> w341
              tunnel: w340 -> [_ _]
              tunnel: w338 -> [w346 _]
              tunnel: w336 -> [w342 _]
              frame False {
                n149 = Greater?(x=w346, y=765.0) -> (0:w343:bool)
                n150 = case shown="True" w343 {
                  tunnel: [w347 767] -> w344
                  tunnel: w342 -> [w347 _]
                  frame False {
                  }
                  frame True {
                  }
                }
              }
              frame True {
              }
            }
          }
        }
      }
    }
    "Fly real-time location 2" <- w137
    "max index(es) of difference 2" <- w137
    n151 = case shown="True" "Fly presence?" {
      tunnel: w301 -> [_ w411]
      tunnel: [0 w410] -> w300
      tunnel: w301 -> [_ w404]
      tunnel: w301 -> [_ w403]
      tunnel: w186 -> [_ w402]
      tunnel: w186 -> [_ w401]
      frame False {
      }
      frame True {
        n152 = Less?(x=w404, y=5.0) -> (x < y?=w407:bool)
        n153 = Greater?(x=w404, y=765.0) -> (0:w405:bool)
        n154 = Or(x=w405, y=w407) -> (x .or. y?=w409:bool)
        n155 = case shown="True" w409 {
          tunnel: w411 -> [w412 w418]
          tunnel: [w412 w419] -> w410
          tunnel: w403 -> [_ w413]
          tunnel: w402 -> [_ w416]
          tunnel: w401 -> [_ w414]
          frame False {
          }
          frame True {
            n156 = Greater?(x=w413, y=765.0) -> (0:w415:bool)
            n157 = case shown="False" w415 {
              tunnel: [w422 767] -> w419
              tunnel: w418 -> [_ _]
              tunnel: w416 -> [w424 _]
              tunnel: w414 -> [w420 _]
              frame False {
                n158 = Greater?(x=w424, y=765.0) -> (0:w421:bool)
                n159 = case shown="True" w421 {
                  tunnel: [w425 767] -> w422
                  tunnel: w420 -> [w425 _]
                  frame False {
                  }
                  frame True {
                  }
                }
              }
              frame True {
              }
            }
          }
        }
      }
    }
    "max index(es) of difference" <- w300
    "Fly real-time location" <- w300
    n160 = And(x=w104, y=w103) -> (x .and. y?=w102:bool)
    n161 = Not(x=w102) -> (.not. x?=w101:bool)
    n162 = Boolean To (0,1)(Boolean=w101) -> (0, 1=→"Laser ON/OFF? 2":i16)
    n163 = Build Array(w300, w131, w96, w153, w108, w94) -> (w299:dbl[])
    n164 = Build Array(w137, w133, w96, w194, w109, w94) -> (w172:dbl[])
    n165 = call "Convert to Dynamic Data"("Array"=w299) -> ("Dynamic Data Type"=w298:dynamicdata)  [unwired: 3 in]
    n166 = TDMS Write(0:w140, 5:"Measured Data" ("group name"), 7:string[] ["Fly_position", "Fly_transient_speed", "Laser_status", "Integral of subtraction data", "Center_of_mass", "Iteration Duration(prev)"] ("channel names"), 9:w298) -> (4:w295:refnum<k34>)  [unwired: 2 in, 3 out]
    n167 = call "Convert to Dynamic Data2"("Array"=w172) -> ("Dynamic Data Type"=w173:dynamicdata)  [unwired: 3 in]
    n168 = TDMS Write(0:w139, 5:"Measured Data" ("group name"), 7:string[] ["Fly_position", "Fly_transient_speed", "Laser_status", "Integral of subtraction data", "Center_of_mass", "Iteration Duration(prev)"] ("channel names"), 9:w173) -> (4:w171:refnum<k34>)  [unwired: 2 in, 3 out]
    n169 = node-c288() -> ()  [unwired: 1 in, 1 out]
  }
  n170 = node-c288(w72) -> ()  [unwired: 1 out]
  n171 = TDMS Close(11:w7) -> ()  [unwired: 1 in, 2 out]
  n172 = TDMS Close(11:w9) -> ()  [unwired: 1 in, 2 out]
  n173 = xnode ("Close FPGA VI Reference")("FPGA VI Reference In"=w58) -> ()  [unwired: 1 in, 1 out]
  n174 = TDMS Close(11:w51) -> ()  [unwired: 1 in, 2 out]
  n175 = TDMS Close(11:w57) -> ()  [unwired: 1 in, 2 out]
